vi "MultiOpto_Host.vi"() -> ()   [LabVIEW 2018]
uses:
  <instrlib>/niDMM/nidmm.llb/niDMM Resolution in Digits.ctl
  <instrlib>/niDMM/nidmm.llb/niDMM Function.ctl
  <instrlib>/niDCPower/nidcpower.llb/niDCPower Measurement Type.ctl
  <instrlib>/niDMM/nidmm.llb/niDMM Configure Measurement Digits.vi
  <instrlib>/niScope/Configure/Trigger/niScope Configure Trigger Window.vi
  <instrlib>/niScope/Acquire/Fetch/niScope Multi Fetch Cluster.vi
  <instrlib>/niScope/Acquire/Fetch/niScope Fetch.vi
panel:
  in  "Full Log Path":path=path "D:/NI LabVIEW/MultiOpto/Full Log"
  in  "Full Log Wait":u32=200
  in  "NI DMM 1":refnum<k15>="PXI1Slot6_3"
  in  "NI DMM 2":refnum<k15>="PXI1Slot6_3"
  in  "Ophir 2 Tab":enum32{"Ophir 2", "System Panel"}(tab)
  out "Ophir 2 Initialization":bool caption="Initialization"
  in  "Ophir 2 Clear":bool caption="Clear"
  out "Ophir 2 MAX":dbl caption="MAX" format="%#_4g"
  out "Ophir 2 Optical Power":dbl caption="Optical Power" format="%#_4g"
  out "Ophir 2 Over Range":bool caption="Over Range"
  out "Ophir 2 Char":dbl(graph)=6.67426339573744e-05
  in  "Ophir 2 units":string(combo)="1000" caption="Units"
  in  "Ophir 2 Info":u16(ring)=1 caption="Info" items=["Device : JUNO; s/n:903794", "Head : PD300-IRG-v1; s/n:908004"]
  in  "Ophir 2 Wait":u32=100 caption="Wait"
  out "Ophir 2 error out":errorcluster caption="error out"
  out "Ophir 2 dup Visa Session":refnum<visa-resource-name>="USB0::0x0BD3::0x0777::NI-VISA-10003::RAW" caption="dup Visa Session"
  in  "Ophir 2 GPIB Address (10)":string="10" caption="GPIB Address (10)"
  in  "Ophir 2 Select Communication Protocol":u16(ring) caption="Select Communication Protocol" items=["USB", "RS232", "GPIB"]
  in  "Ophir 2 usb channel":i16 caption="usb channel"
  in  "Ophir 2 Baud Rate (3:9600)":i16(ring)=3 caption="Baud Rate (3:9600)" items=["300", "1200", "4800", "9600", "19200", "38400"]
  in  "Ophir 2 Port Number (default 2)":i16=2 caption="Port Number (default 2)" min=0 max=20
  in  "Ophir 2 error in (no error)":errorcluster caption="error in (no error)"
  out "Ophir 2 Status":bool caption="Status"
  out "Ophir 2 Real Optical Power":dbl format="%.3e"
  in  "Ophir 1 Tab":enum32{"Ophir 1", "System Panel"}(tab)
  out "Ophir 1 Initialization":bool caption="Initialization"
  in  "Ophir 1 units":string(combo)="1000" caption="Units"
  out "Ophir 1 Char":dbl(graph)=6.67426339573744e-05
  out "Ophir 1 Over Range":bool caption="Over Range"
  out "Ophir 1 Optical Power":dbl caption="Optical Power" format="%#_4g"
  out "Ophir 1 MAX":dbl caption="MAX" format="%#_4g"
  in  "Ophir 1 Clear":bool caption="Clear"
  in  "Ophir 1 Info":u16(ring)=1 caption="Info" items=["Device : JUNO; s/n:903795", "Head : PD300R-IR   ; s/n:873888"]
  in  "Ophir 1 Wait":u32=100 caption="Wait"
  in  "Ophir 1 error in (no error)":errorcluster caption="error in (no error)"
  out "Ophir 1 error out":errorcluster caption="error out"
  in  "Ophir 1 Select Communication Protocol":u16(ring) caption="Select Communication Protocol" items=["USB", "RS232", "GPIB"]
  in  "Ophir 1 usb channel":i16 caption="usb channel"
  in  "Ophir 1 Port Number (default 2)":i16=1 caption="Port Number (default 2)" min=0 max=20
  in  "Ophir 1 Baud Rate (3:9600)":i16(ring)=3 caption="Baud Rate (3:9600)" items=["300", "1200", "4800", "9600", "19200", "38400"]
  in  "Ophir 1 GPIB Address (10)":string="10" caption="GPIB Address (10)"
  out "Ophir 1 dup Visa Session":refnum<visa-resource-name>="USB0::0x0BD3::0x0777::NI-VISA-10003::RAW" caption="dup Visa Session"
  out "Ophir 1 Status":bool caption="Status"
  out "Ophir 1 Real Optical Power":dbl format="%.3e"
  out "Образец №":string
  in  "NI DMM 2 Tab":enum32{"Ampermeter", "Ohmmeter", "System Panel"}(tab)
  out "NI DMM 2 Current":dbl caption="Current" format="%_4g"
  out "NI DMM 2 Current Char":dbl(graph)=6.67426339573744e-05
  in  "NI DMM 2 Ampermeter path":path=path "D:/NI LabVIEW/MultiOpto/NI DMM 2" caption="NI DMM 2 Path"
  in  "NI DMM 2 units":string(combo)="1" caption="Units"
  in  "NI DMM 2 Current Range":string(combo)="-1" caption="Range"
  in  "NI DMM 2 Current Wait":u32=100 caption="Wait"
  in  "NI DMM 2 Ohmmeter path":path=path "D:/NI LabVIEW/MultiOpto/NI DMM 2" caption="Ohmmeter Path"
  out "NI DMM 2 Resistance":dbl caption="Resistance" format="%_4g"
  out "NI DMM 2 Resistance Char":dbl(graph)=6.67426339573744e-05
  in  "NI DMM 2 Resistance units":string(combo)="1" caption="Units"
  in  "NI DMM 2 Resistance Range":string(combo)="-1" caption="Range"
  in  "NI DMM 2 Resistance Wait":u32=100 caption="Wait"
  out "NI DMM 2 Status":bool
  out "NI DMM 2 Current output file":refnum<file>
  out "NI DMM 2error out":errorcluster
  in  "NI DMM 2 error in":errorcluster
  out "NI DMM 2 Option Return":enum32{"Ampermeter button", "Ohmmeter button"}(ring)
  out "NI DMM 2 Resistance output file":refnum<file>
  in  "NI DMM 1 Tab":enum32{"Ampermeter", "Ohmmeter", "System Panel"}(tab)
  out "NI DMM 1 Current Char":dbl(graph)=6.67426339573744e-05
  out "NI DMM 1 Current":dbl caption="Current" format="%_4g"
  in  "NI DMM 1 Ampermeter path":path=path "D:/NI LabVIEW/MultiOpto/NI DMM 1" caption="Ampermeter Path"
  in  "NI DMM 1 units":string(combo)="1" caption="Units"
  in  "NI DMM 1 Current Range":string(combo)="-1" caption="Range"
  in  "NI DMM 1 Current Wait":u32=100 caption="Wait"
  in  "NI DMM 1 Ohmmeter path":path=path "D:/NI LabVIEW/MultiOpto/NI DMM 1" caption="Ohmmeter Path"
  out "NI DMM 1 Resistance":dbl caption="Resistance" format="%_6g"
  out "NI DMM 1 Resistance Char":dbl(graph)=6.67426339573744e-05
  in  "NI DMM 1 Resistance units":string(combo)="1" caption="Units"
  in  "NI DMM 1 Resistance Range":string(combo)="-1" caption="Range"
  in  "NI DMM 1 Resistance Wait":u32=100 caption="Wait"
  out "NI DMM 1 Status":bool
  out "NI DMM 1 Current output file":refnum<file>
  out "NI DMM 1 error out":errorcluster
  in  "NI DMM 1 error in":errorcluster
  out "NI DMM 1 Option Return":enum32{"Ampermeter button", "Ohmmeter button"}(ring)
  out "NI DMM 1 Resistance output file":refnum<file>
  out "SEL":bool
  out "SEU":bool caption="SEL"
  in  "NI Scope Tab":enum32{"NI Scope", "System Panel"}(tab)
  in  "vertical range":dbl=2.0 caption="Vertical Range" format="%.2f"
  out "SEU Last Level":dbl
  out "RealTime Waveform":T1(graph) caption="PC_MON Waveform"
  out "SEU Waveform":T1(graph) caption="SHUTDOWN Waveform"
  out "SEU_Counter":u32 caption="SEU counter"
  out "SEU_warning":bool caption="Find SEL"
  in  "Low Level":dbl=0.35 format="%.2f"
  in  "High Level":dbl=0.65 format="%.2f"
  in  "NI Scope":refnum<k15>="PXI1Slot5_2" caption="Scope"
  in  "AC/DC/Groun":i32(ring)=1 items=["AC", "DC", "Ground"]
  in  "Trigger Source":string(combo)="0"
  in  "SEU path":path=path "D:/NI LabVIEW/MultiOpto/SEU" caption="SEU Path"
  in  "Channel for SEU":T2(radio)
  out "SEU output file refnum":refnum<file>
  out "NI Scope Status":bool
  out "NI Scope error out":errorcluster
  in  "NI Scope error in":errorcluster
  in  "STOP":bool
  in  "DC Power Tab":enum32{"DC-Power", "System Panel"}(tab)
  out "P2 CH1_warning":bool caption="VCC_warning"
  out "P2 CH1_counter":u32 caption="VCC_counter"
  in  "P2 CH1_selcur, A":dbl=0.2 caption="current limit" format="%_6p"
  in  "P2 CH1 Used":bool
  in  "P2 CH1":bool
  out "P2 CH1_char":dbl(graph)=4.1881856349625015e-07
  in  "P2 CH1, V":dbl=4.9 caption="voltage level" format="%_6p"
  out "P2 CH1_cur, A":dbl caption="measurement" format="%_6g"
  in  "P2 CH1_curlim, A":dbl=0.015 caption="current limit" format="%_6p"
  in  "P1 CH0_selcur, A":dbl=0.2 caption="current limit" format="%_6p"
  in  "P1 CH1_selcur, A":dbl=0.2 caption="current limit" format="%_6p"
  in  "P2 CH0_selcur, A":dbl=0.2 caption="current limit" format="%_6p"
  out "P2 CH0_counter":u32 caption="VCC_counter"
  out "P2 CH0_warning":bool caption="VCC_warning"
  out "P1 CH1_counter":u32 caption="VCC_counter"
  out "P1 CH1_warning":bool caption="VCC_warning"
  out "P1 CH0_counter":u32 caption="VCC_counter"
  out "P1 CH0_warning":bool caption="VCC_warning"
  in  "P2 CH0":bool
  in  "P1 CH1":bool
  in  "P1 CH0":bool
  in  "P2 CH0_curlim, A":dbl=0.015 caption="current limit" format="%_6p"
  out "P2 CH0_cur, A":dbl caption="measurement" format="%_6g"
  in  "P2 CH0, V":dbl=2.5 caption="voltage level" format="%_6p"
  out "P2 CH0_char":dbl(graph)=8.408429577071082e-05
  in  "P1 CH1_curlim, A":dbl=0.015 caption="current limit" format="%_6p"
  out "P1CH1_cur, A":dbl caption="measurement" format="%_6g"
  in  "P1 CH1, V":dbl=2.5 caption="voltage level" format="%_6p"
  out "P1 CH1_char":dbl(graph)=6.336785656464814e-07
  in  "P1 CH0_curlim, A":dbl=0.015 caption="current limit" format="%_6p"
  out "P1 CH0_cur, A":dbl caption="measurement" format="%_6g"
  in  "P1 CH0, V":dbl=2.5 caption="voltage level" format="%_6p"
  out "P1 CH0_char":dbl(graph)=8.030591065176734e-05
  in  "POWER 2 (CH0, CH1)":refnum<k15>="PXI1Slot3_3" caption="PRBS"
  in  "POWER 1 (CH0, CH1)":refnum<k15>="PXI1Slot2_2" caption="VСС_+5"
  in  "P1 CH0 Used":bool
  in  "P2 CH0 Used":bool
  in  "P1 CH1 Used":bool
  in  "SIM_SEL":bool
  in  "SEL Time Cycle":u32=100
  in  "SEL path":path=path "D:/NI LabVIEW/MultiOpto/SEL" caption="SEL Path"
  out "Power OFF":bool
  in  "Считать SIM_SEL":bool
  out "Ready Status":bool
  out "DC Power 2 error out":errorcluster
  out "DC Power 1 error out":errorcluster
  out "SEL output file refnum":refnum<file>
  # "Че там?"
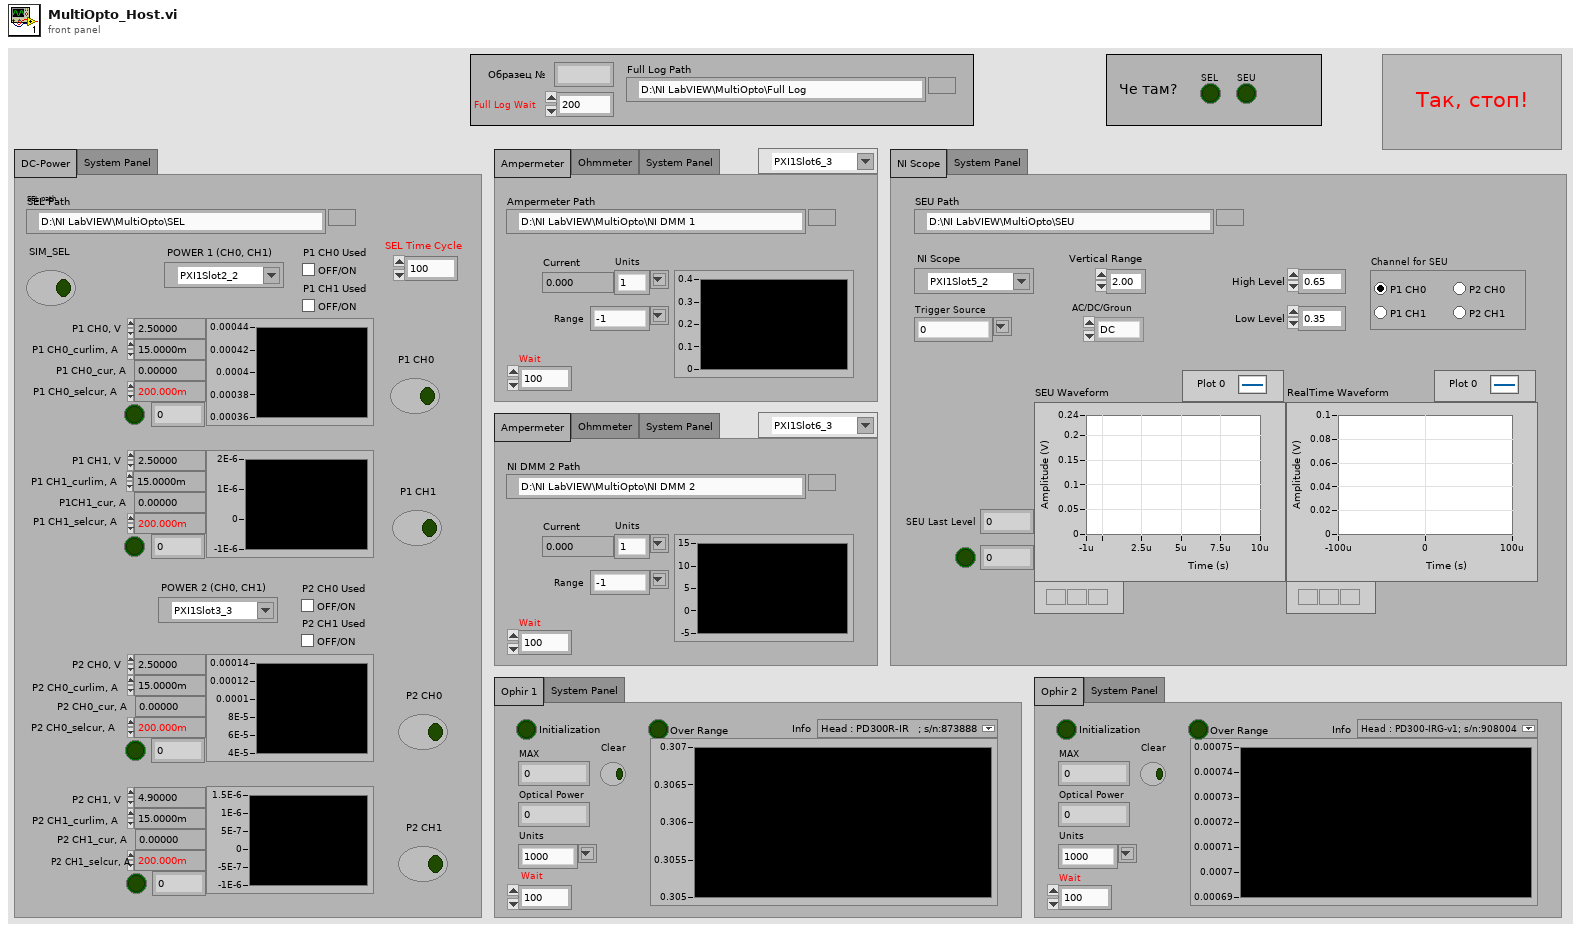
[diagram p1: front panel]
types:
  T1 = cluster{"relativeInitialX":dbl, "xIncrement":dbl, "wfm":dbl[]}[]
  T2 = enum32{"Radio Selection P1 CH0", "Radio Selection P1 CH1", "Radio Selection P2 CH0", "Radio Selection P2 CH1"}
  T3 = enum8{"Enabled", "Disabled", "Disabled and Grayed Out"}
  T4 = enum16{"open", "replace", "create", "open or create", "replace or create", "replace or create with confirmation"}
  T5 = typedef "niDMM Function.ctl" = enum16{"DC Volts", "AC Volts", "DC Current", "AC Current", "2-wire Resistance", "4-wire Resistance", "Diode", "Frequency", "Period", "AC Volts DC Coupled", "Capacitance", "Inductance", "Temperature"}
  T6 = typedef "niDMM Resolution in Digits.ctl" = dbl
  T7 = typedef "niDCPower Measurement Type.ctl" = i32
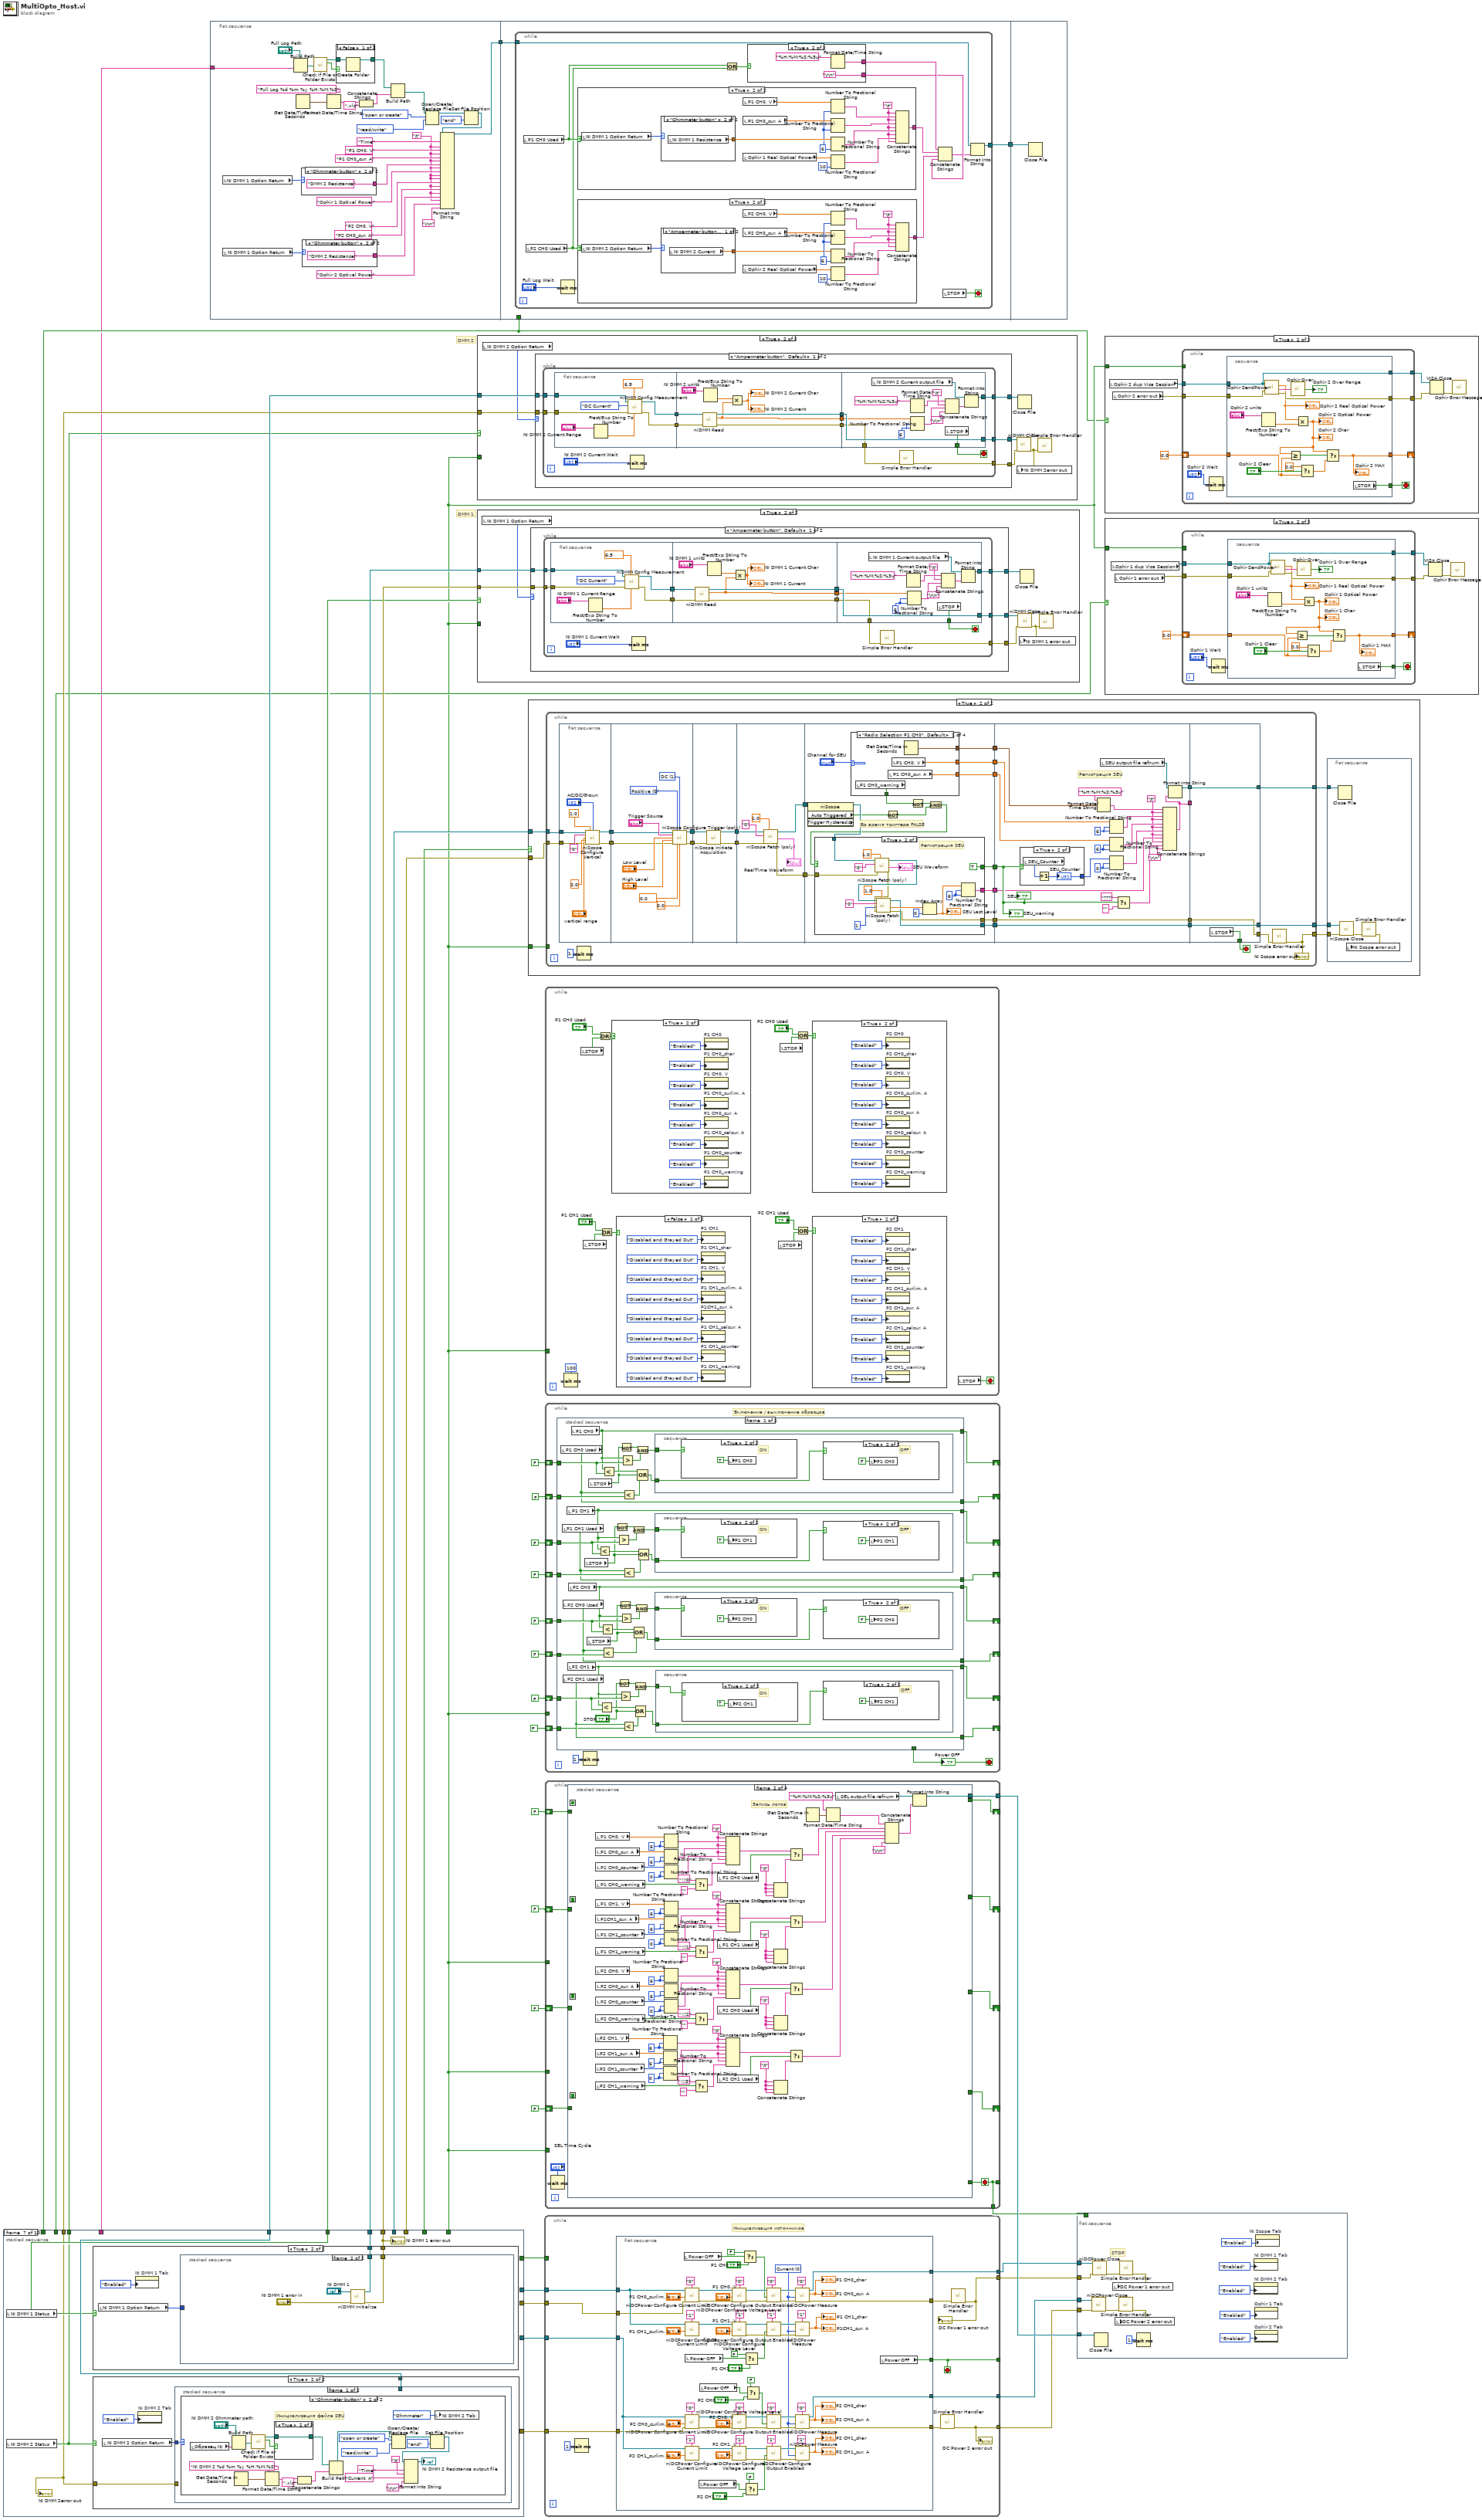
[diagram p0: block diagram]
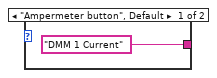
[diagram p2: hidden frame]
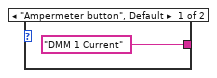
[diagram p3: hidden frame]
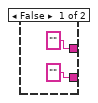
[diagram p5: hidden frame]
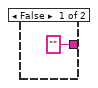
[diagram p6: hidden frame]
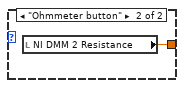
[diagram p7: hidden frame]
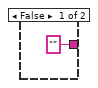
[diagram p8: hidden frame]
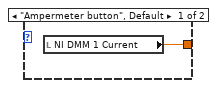
[diagram p9: hidden frame]
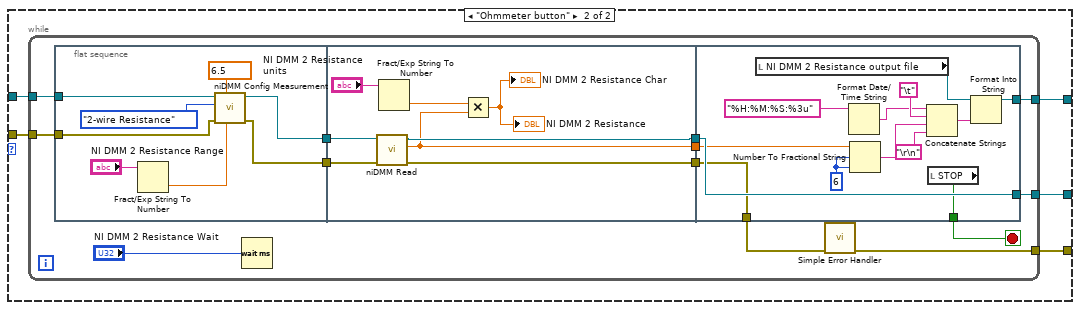
[diagram p13: hidden frame]
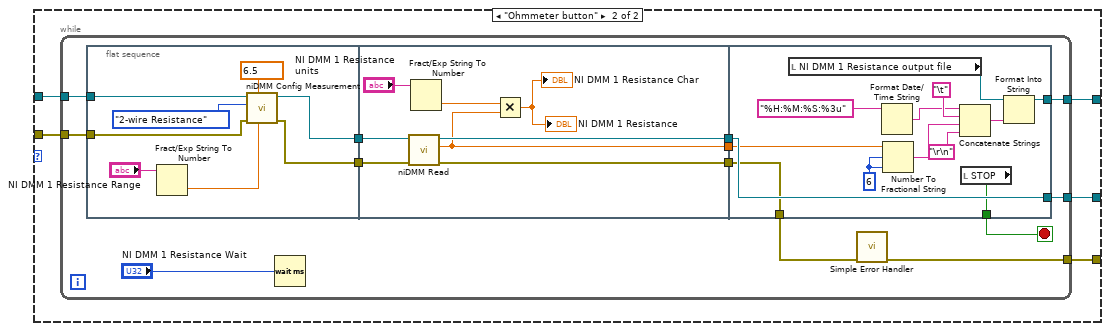
[diagram p15: hidden frame]
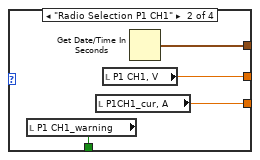
[diagram p17: hidden frame]
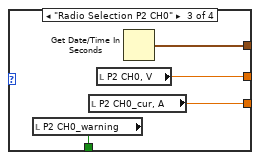
[diagram p18: hidden frame]
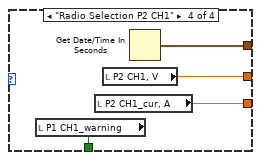
[diagram p19: hidden frame]
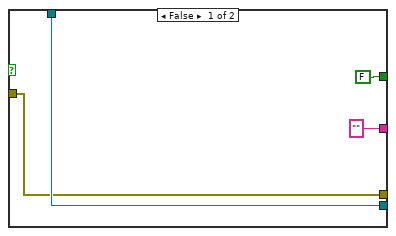
[diagram p20: hidden frame]
diagram:
  # "DMM 2"
  # "DMM 1"
  n1 = stacked-sequence {
    tunnel: [_ _ _ _ w165 _ _ _ _ _] -> w23
    tunnel: [_ _ _ _ w164 _ _ _ _ _] -> w22
    tunnel: [_ _ _ _ w163 _ _ _ _ _] -> w18
    tunnel: [_ _ _ _ w162 _ _ _ _ _] -> w17
    tunnel: [_ _ _ _ _ _ _ _ _ w412] -> w16
    tunnel: [_ _ _ _ _ _ _ _ _ w412] -> w3
    tunnel: [_ _ _ _ _ w178 _ _ _ _] -> w15
    tunnel: [_ _ _ _ _ _ w234 _ _ _] -> w14
    tunnel: [_ _ _ _ _ _ w237 _ _ _] -> w13
    tunnel: [_ _ _ _ _ w177 _ _ _ _] -> w12
    tunnel: [_ _ _ _ _ _ w233 _ _ _] -> w11
    tunnel: [_ _ _ _ _ _ w232 _ _ _] -> w10
    tunnel: [_ _ _ _ _ w176 _ _ _ _] -> w9
    tunnel: [_ _ _ _ _ _ w236 _ _ _] -> w8
    tunnel: [_ _ _ _ _ _ w235 _ _ _] -> w7
    tunnel: [_ _ _ _ _ _ _ w366 _ _] -> w6
    tunnel: [_ _ _ _ _ _ _ _ w389 _] -> w2
    tunnel: [_ _ w114 _ _ _ _ _ _ _] -> w1
    frame #0 {
      w39 = FALSE
      w41 = FALSE ("NI Scope Status")
      w44 = u32 0 ("SEU_Counter")
      w40 = FALSE ("STOP")
      # "Начальная конфигурация переменных"
      n2 = local write "Ophir 2 Over Range"(w39) -> ()
      n3 = local write "Ophir 1 Over Range"(w39) -> ()
      n4 = local write "Ophir 1 Initialization"(w39) -> ()
      n5 = local write "Ophir 2 Initialization"(w39) -> ()
      n6 = local write "Ophir 1 Clear"(w39) -> ()
      n7 = local write "Ophir 2 Clear"(w39) -> ()
      n8 = local write "STOP"(w40) -> ()
      n9 = local write "P1 CH0"(w40) -> ()
      n10 = local write "P1 CH1"(w40) -> ()
      n11 = local write "P2 CH0"(w40) -> ()
      n12 = local write "P2 CH1"(w40) -> ()
      n13 = local write "Power OFF"(w40) -> ()
      n14 = local write "P1 CH0 Used"(w40) -> ()
      n15 = local write "P1 CH1 Used"(w40) -> ()
      n16 = local write "P2 CH0 Used"(w40) -> ()
      n17 = local write "P2 CH1 Used"(w40) -> ()
      n18 = local write "Считать SIM_SEL"(w40) -> ()
      n19 = local write "SEL"(w40) -> ()
      n20 = local write "SEU"(w40) -> ()
      n21 = local write "SEU_warning"(w40) -> ()
      n22 = local write "P1 CH0_warning"(w40) -> ()
      n23 = local write "P1 CH1_warning"(w40) -> ()
      n24 = local write "P2 CH0_warning"(w40) -> ()
      n25 = local write "P2 CH1_warning"(w40) -> ()
      n26 = local write "SEU_warning"(w40) -> ()
      n27 = local write "SEU Last Level"(0.0 ("SEU Level")) -> ()
      n28 = local write "SEU_Counter"(w44) -> ()
      n29 = local write "P1 CH0_counter"(w44) -> ()
      n30 = local write "P1 CH1_counter"(w44) -> ()
      n31 = local write "P2 CH0_counter"(w44) -> ()
      n32 = local write "P2 CH1_counter"(w44) -> ()
      n33 = local write "Образец №"("" ("Образец №")) -> ()
      n34 = local write "Ready Status"(FALSE ("Ready Status")) -> ()
      n35 = local write "NI Scope Status"(w41) -> ()
      n36 = local write "NI DMM 2 Status"(w41) -> ()
      n37 = local write "NI DMM 1 Status"(w41) -> ()
      n38 = local write "Ophir 1 Status"(w41) -> ()
      n39 = local write "Ophir 2 Status"(w41) -> ()
    }
    frame #1 {
      n40 = stacked-sequence {
        frame #0 {
          n41 = local read "P1 CH0 Used"() -> (w46:bool)
          n42 = case shown="False" w46 {
            frame False {
              n43 = property on="P1 CH0" class="Bool (strict)"("DisabledEnum"=T3."Disabled and Grayed Out" ("Disabled")) -> ()  [unwired: 2 in, 2 out]
              n44 = property on="P1 CH0_char" class="WFChart (strict)"("DisabledEnum"=T3."Disabled and Grayed Out" ("Disabled")) -> ()  [unwired: 2 in, 2 out]
              n45 = property on="P1 CH0, V" class="DigNum (strict)"("DisabledEnum"=T3."Disabled and Grayed Out" ("Disabled")) -> ()  [unwired: 2 in, 2 out]
              n46 = property on="P1 CH0_curlim, A" class="DigNum (strict)"("DisabledEnum"=T3."Disabled and Grayed Out" ("Disabled")) -> ()  [unwired: 2 in, 2 out]
              n47 = property on="P1 CH0_cur, A" class="DigNum (strict)"("DisabledEnum"=T3."Disabled and Grayed Out" ("Disabled")) -> ()  [unwired: 2 in, 2 out]
              n48 = property on="P1 CH0_selcur, A" class="DigNum (strict)"("DisabledEnum"=T3."Disabled and Grayed Out" ("Disabled")) -> ()  [unwired: 2 in, 2 out]
              n49 = property on="P1 CH0_counter" class="DigNum (strict)"("DisabledEnum"=T3."Disabled and Grayed Out" ("Disabled")) -> ()  [unwired: 2 in, 2 out]
              n50 = property on="P1 CH0_warning" class="Bool (strict)"("DisabledEnum"=T3."Disabled and Grayed Out" ("Disabled")) -> ()  [unwired: 2 in, 2 out]
            }
            frame True {
              n51 = property on="P1 CH0" class="Bool (strict)"("DisabledEnum"=T3."Enabled" ("Disabled")) -> ()  [unwired: 2 in, 2 out]
              n52 = property on="P1 CH0_char" class="WFChart (strict)"("DisabledEnum"=T3."Enabled" ("Disabled")) -> ()  [unwired: 2 in, 2 out]
              n53 = property on="P1 CH0, V" class="DigNum (strict)"("DisabledEnum"=T3."Enabled" ("Disabled")) -> ()  [unwired: 2 in, 2 out]
              n54 = property on="P1 CH0_curlim, A" class="DigNum (strict)"("DisabledEnum"=T3."Enabled" ("Disabled")) -> ()  [unwired: 2 in, 2 out]
              n55 = property on="P1 CH0_cur, A" class="DigNum (strict)"("DisabledEnum"=T3."Enabled" ("Disabled")) -> ()  [unwired: 2 in, 2 out]
              n56 = property on="P1 CH0_selcur, A" class="DigNum (strict)"("DisabledEnum"=T3."Enabled" ("Disabled")) -> ()  [unwired: 2 in, 2 out]
              n57 = property on="P1 CH0_counter" class="DigNum (strict)"("DisabledEnum"=T3."Enabled" ("Disabled")) -> ()  [unwired: 2 in, 2 out]
              n58 = property on="P1 CH0_warning" class="Bool (strict)"("DisabledEnum"=T3."Enabled" ("Disabled")) -> ()  [unwired: 2 in, 2 out]
            }
          }
        }
        frame #1 {
          n59 = local read "P1 CH1 Used"() -> (w63:bool)
          n60 = case shown="False" w63 {
            frame False {
              n61 = property on="P1 CH1" class="Bool (strict)"("DisabledEnum"=T3."Disabled and Grayed Out" ("Disabled")) -> ()  [unwired: 2 in, 2 out]
              n62 = property on="P1 CH1_char" class="WFChart (strict)"("DisabledEnum"=T3."Disabled and Grayed Out" ("Disabled")) -> ()  [unwired: 2 in, 2 out]
              n63 = property on="P1 CH1, V" class="DigNum (strict)"("DisabledEnum"=T3."Disabled and Grayed Out" ("Disabled")) -> ()  [unwired: 2 in, 2 out]
              n64 = property on="P1 CH1_curlim, A" class="DigNum (strict)"("DisabledEnum"=T3."Disabled and Grayed Out" ("Disabled")) -> ()  [unwired: 2 in, 2 out]
              n65 = property on="P1CH1_cur, A" class="DigNum (strict)"("DisabledEnum"=T3."Disabled and Grayed Out" ("Disabled")) -> ()  [unwired: 2 in, 2 out]
              n66 = property on="P1 CH1_selcur, A" class="DigNum (strict)"("DisabledEnum"=T3."Disabled and Grayed Out" ("Disabled")) -> ()  [unwired: 2 in, 2 out]
              n67 = property on="P1 CH1_counter" class="DigNum (strict)"("DisabledEnum"=T3."Disabled and Grayed Out" ("Disabled")) -> ()  [unwired: 2 in, 2 out]
              n68 = property on="P1 CH1_warning" class="Bool (strict)"("DisabledEnum"=T3."Disabled and Grayed Out" ("Disabled")) -> ()  [unwired: 2 in, 2 out]
            }
            frame True {
              n69 = property on="P1 CH1" class="Bool (strict)"("DisabledEnum"=T3."Enabled" ("Disabled")) -> ()  [unwired: 2 in, 2 out]
              n70 = property on="P1 CH1_char" class="WFChart (strict)"("DisabledEnum"=T3."Enabled" ("Disabled")) -> ()  [unwired: 2 in, 2 out]
              n71 = property on="P1 CH1, V" class="DigNum (strict)"("DisabledEnum"=T3."Enabled" ("Disabled")) -> ()  [unwired: 2 in, 2 out]
              n72 = property on="P1 CH1_curlim, A" class="DigNum (strict)"("DisabledEnum"=T3."Enabled" ("Disabled")) -> ()  [unwired: 2 in, 2 out]
              n73 = property on="P1CH1_cur, A" class="DigNum (strict)"("DisabledEnum"=T3."Enabled" ("Disabled")) -> ()  [unwired: 2 in, 2 out]
              n74 = property on="P1 CH1_selcur, A" class="DigNum (strict)"("DisabledEnum"=T3."Enabled" ("Disabled")) -> ()  [unwired: 2 in, 2 out]
              n75 = property on="P1 CH1_counter" class="DigNum (strict)"("DisabledEnum"=T3."Enabled" ("Disabled")) -> ()  [unwired: 2 in, 2 out]
              n76 = property on="P1 CH1_warning" class="Bool (strict)"("DisabledEnum"=T3."Enabled" ("Disabled")) -> ()  [unwired: 2 in, 2 out]
            }
          }
        }
        frame #2 {
          n77 = local read "P2 CH0 Used"() -> (w80:bool)
          n78 = case shown="False" w80 {
            frame False {
              n79 = property on="P2 CH0" class="Bool (strict)"("DisabledEnum"=T3."Disabled and Grayed Out" ("Disabled")) -> ()  [unwired: 2 in, 2 out]
              n80 = property on="P2 CH0_char" class="WFChart (strict)"("DisabledEnum"=T3."Disabled and Grayed Out" ("Disabled")) -> ()  [unwired: 2 in, 2 out]
              n81 = property on="P2 CH0, V" class="DigNum (strict)"("DisabledEnum"=T3."Disabled and Grayed Out" ("Disabled")) -> ()  [unwired: 2 in, 2 out]
              n82 = property on="P2 CH0_curlim, A" class="DigNum (strict)"("DisabledEnum"=T3."Disabled and Grayed Out" ("Disabled")) -> ()  [unwired: 2 in, 2 out]
              n83 = property on="P2 CH0_cur, A" class="DigNum (strict)"("DisabledEnum"=T3."Disabled and Grayed Out" ("Disabled")) -> ()  [unwired: 2 in, 2 out]
              n84 = property on="P2 CH0_selcur, A" class="DigNum (strict)"("DisabledEnum"=T3."Disabled and Grayed Out" ("Disabled")) -> ()  [unwired: 2 in, 2 out]
              n85 = property on="P2 CH0_counter" class="DigNum (strict)"("DisabledEnum"=T3."Disabled and Grayed Out" ("Disabled")) -> ()  [unwired: 2 in, 2 out]
              n86 = property on="P2 CH0_warning" class="Bool (strict)"("DisabledEnum"=T3."Disabled and Grayed Out" ("Disabled")) -> ()  [unwired: 2 in, 2 out]
            }
            frame True {
              n87 = property on="P2 CH0" class="Bool (strict)"("DisabledEnum"=T3."Enabled" ("Disabled")) -> ()  [unwired: 2 in, 2 out]
              n88 = property on="P2 CH0_char" class="WFChart (strict)"("DisabledEnum"=T3."Enabled" ("Disabled")) -> ()  [unwired: 2 in, 2 out]
              n89 = property on="P2 CH0, V" class="DigNum (strict)"("DisabledEnum"=T3."Enabled" ("Disabled")) -> ()  [unwired: 2 in, 2 out]
              n90 = property on="P2 CH0_curlim, A" class="DigNum (strict)"("DisabledEnum"=T3."Enabled" ("Disabled")) -> ()  [unwired: 2 in, 2 out]
              n91 = property on="P2 CH0_cur, A" class="DigNum (strict)"("DisabledEnum"=T3."Enabled" ("Disabled")) -> ()  [unwired: 2 in, 2 out]
              n92 = property on="P2 CH0_selcur, A" class="DigNum (strict)"("DisabledEnum"=T3."Enabled" ("Disabled")) -> ()  [unwired: 2 in, 2 out]
              n93 = property on="P2 CH0_counter" class="DigNum (strict)"("DisabledEnum"=T3."Enabled" ("Disabled")) -> ()  [unwired: 2 in, 2 out]
              n94 = property on="P2 CH0_warning" class="Bool (strict)"("DisabledEnum"=T3."Enabled" ("Disabled")) -> ()  [unwired: 2 in, 2 out]
            }
          }
        }
        frame #3 {
          n95 = local read "P2 CH1 Used"() -> (w97:bool)
          n96 = case shown="False" w97 {
            frame False {
              n97 = property on="P2 CH1" class="Bool (strict)"("DisabledEnum"=T3."Disabled and Grayed Out" ("Disabled")) -> ()  [unwired: 2 in, 2 out]
              n98 = property on="P2 CH1_char" class="WFChart (strict)"("DisabledEnum"=T3."Disabled and Grayed Out" ("Disabled")) -> ()  [unwired: 2 in, 2 out]
              n99 = property on="P2 CH1, V" class="DigNum (strict)"("DisabledEnum"=T3."Disabled and Grayed Out" ("Disabled")) -> ()  [unwired: 2 in, 2 out]
              n100 = property on="P2 CH1_curlim, A" class="DigNum (strict)"("DisabledEnum"=T3."Disabled and Grayed Out" ("Disabled")) -> ()  [unwired: 2 in, 2 out]
              n101 = property on="P2 CH1_cur, A" class="DigNum (strict)"("DisabledEnum"=T3."Disabled and Grayed Out" ("Disabled")) -> ()  [unwired: 2 in, 2 out]
              n102 = property on="P2 CH1_selcur, A" class="DigNum (strict)"("DisabledEnum"=T3."Disabled and Grayed Out" ("Disabled")) -> ()  [unwired: 2 in, 2 out]
              n103 = property on="P2 CH1_counter" class="DigNum (strict)"("DisabledEnum"=T3."Disabled and Grayed Out" ("Disabled")) -> ()  [unwired: 2 in, 2 out]
              n104 = property on="P2 CH1_warning" class="Bool (strict)"("DisabledEnum"=T3."Disabled and Grayed Out" ("Disabled")) -> ()  [unwired: 2 in, 2 out]
            }
            frame True {
              n105 = property on="P2 CH1" class="Bool (strict)"("DisabledEnum"=T3."Enabled" ("Disabled")) -> ()  [unwired: 2 in, 2 out]
              n106 = property on="P2 CH1_char" class="WFChart (strict)"("DisabledEnum"=T3."Enabled" ("Disabled")) -> ()  [unwired: 2 in, 2 out]
              n107 = property on="P2 CH1, V" class="DigNum (strict)"("DisabledEnum"=T3."Enabled" ("Disabled")) -> ()  [unwired: 2 in, 2 out]
              n108 = property on="P2 CH1_curlim, A" class="DigNum (strict)"("DisabledEnum"=T3."Enabled" ("Disabled")) -> ()  [unwired: 2 in, 2 out]
              n109 = property on="P2 CH1_cur, A" class="DigNum (strict)"("DisabledEnum"=T3."Enabled" ("Disabled")) -> ()  [unwired: 2 in, 2 out]
              n110 = property on="P2 CH1_selcur, A" class="DigNum (strict)"("DisabledEnum"=T3."Enabled" ("Disabled")) -> ()  [unwired: 2 in, 2 out]
              n111 = property on="P2 CH1_counter" class="DigNum (strict)"("DisabledEnum"=T3."Enabled" ("Disabled")) -> ()  [unwired: 2 in, 2 out]
              n112 = property on="P2 CH1_warning" class="Bool (strict)"("DisabledEnum"=T3."Enabled" ("Disabled")) -> ()  [unwired: 2 in, 2 out]
            }
          }
        }
      }
    }
    frame #2 {
      n113 = call "MultiOpto_Begin.vi"() -> ("NI DMM 2 Status"=→"NI DMM 2 Status":bool, "NI DMM 1 Status"=→"NI DMM 1 Status":bool, "Ophir 2 Status"=→"Ophir 2 Status":bool, "Ophir 1 Status"=→"Ophir 1 Status":bool, "Текущий Образец №"=w114:string, "NI Scope Status"=→"NI Scope Status":bool, "NI DMM 2 option return"=→"NI DMM 2 Option Return":enum32{"Ampermeter button", "Ohmmeter button"}, "NI DMM 1 option return"=→"NI DMM 1 Option Return":enum32{"Ampermeter button", "Ohmmeter button"})  [unwired: 2 in]
      "Образец №" <- w114
    }
    frame #3 {
      w124 = "\t"
      # "Инициализация файла SEL"
      n114 = local read "Образец №"() -> (w143:string)
      n115 = Build Path(base path="SEL path", name or relative path=w143) -> (appended path=w158:path)
      n116 = Get Date/Time In Seconds() -> (seconds since 1Jan1904=w154:timestamp)
      n117 = call <vilib>:"Check if File or Folder Exists.vi"("path"=w158) -> ("file or folder exists?"=w157:bool, "dup path"=w156:path)  [unwired: 8 in, 1 out]
      n118 = Format Date/Time String(time format string (%c)="SEL %d %m %y %H.%M.%S", seconds (now)=w154) -> (date/time string=w153:string)  [unwired: 1 in]
      n119 = case shown="True" w157 {
        tunnel: w156 -> [w160 w161]
        tunnel: [w159 w161] -> w155
        frame False {
          n120 = Create Folder(path (use dialog)=w160) -> (created path=w159:path)  [unwired: 2 in, 2 out]
        }
        frame True {
        }
      }
      n121 = Concatenate Strings(w153, ".xls" ("string")) -> (w150:string)
      n122 = Build Path(base path=w155, name or relative path=w150) -> (appended path=w147:path)
      n123 = Open/Create/Replace File(file path (use dialog)=w147, operation (0:open)=T4."open or create", access (0:read/write)=enum16{"read/write", "read-only", "write-only"}."read/write") -> (refnum out=w146:refnum<file>)  [unwired: 3 in, 2 out]
      n124 = Set File Position(refnum=w146, from (0:start)=enum16{"start", "end", "current"}."end") -> (refnum out=w125:refnum<file>)  [unwired: 2 in, 1 out]
      n125 = Format Into String(initial string=w125, "Time" ("string"), w124, "P1 CH0, V" ("string"), w124, "P1 CH0_cur, A" ("string"), w124, "P1 CH0_counter" ("string"), w124, "!!!0" ("input 7"), w124, "P1 CH1, V" ("string"), w124, "P1 CH1_cur, A" ("string"), w124, "P1 CH1_counter" ("string"), w124, "!!!1" ("input 7"), w124, "P2 CH0, V" ("string"), w124, "P2 CH0_cur, A" ("string"), w124, "P2 CH0_counter" ("string"), w124, "!!!2" ("input 7"), w124, "P2 CH1, V" ("string"), w124, "P2 CH1_cur, A" ("string"), w124, "P2 CH1_counter" ("string"), "!!!3" ("input 7"), "\r\n") -> (resulting string=→"SEL output file refnum":refnum<file>)  [unwired: 2 in, 1 out]
    }
    frame #4 {
      # "Инициализация источника"
      n126 = call <instrlib>:"niDCPower Initialize.vi"("resource name"="POWER 1 (CH0, CH1)") -> ("error out"=w174:errorcluster, "instrument handle out"=w175:refnum<k15>)  [unwired: 3 in, 6 out]
      n127 = call <instrlib>:"niDCPower Initialize.vi"("resource name"="POWER 2 (CH0, CH1)") -> ("error out"=w171:errorcluster, "instrument handle out"=w172:refnum<k15>)  [unwired: 3 in, 6 out]
      n128 = call <instrlib>:"niDCPower Configure Voltage Level.vi"("error in (no error)"=w174, "voltage level"=0.0, "channel name"="0,1", "instrument handle"=w175) -> ("error out"=w163:errorcluster, "instrument handle out"=w165:refnum<k15>)  [unwired: 6 in]
      n129 = call <instrlib>:"niDCPower Configure Voltage Level.vi"("error in (no error)"=w171, "voltage level"=0.0, "channel name"="0,1", "instrument handle"=w172) -> ("error out"=w162:errorcluster, "instrument handle out"=w164:refnum<k15>)  [unwired: 6 in]
    }
    frame #5 {
      n130 = local read "NI Scope Status"() -> (w176:bool)
      n131 = case shown="True" w176 {
        tunnel: [refnum<k15> refnum ("instrument handle out") w184] -> w178
        tunnel: [errorcluster {"status"=FALSE, "code"=0, "source"=""} ("error out") w183] -> w177
        frame False {
          n132 = Wait (ms)(milliseconds to wait=u32 1) -> ()  [unwired: 1 out]
          n133 = property on="NI Scope Tab" class="TabCtl (strict)"("DisabledEnum"=T3."Disabled and Grayed Out" ("Disabled")) -> ()  [unwired: 2 in, 2 out]
        }
        frame True {
          n134 = stacked-sequence {
            tunnel: [_ w216] -> w184
            tunnel: [_ w215] -> w183
            frame #0 {
              w195 = "\t"
              # "Инициализация файла SEU"
              n135 = local read "Образец №"() -> (w200:string)
              n136 = Build Path(base path="SEU path", name or relative path=w200) -> (appended path=w210:path)
              n137 = Get Date/Time In Seconds() -> (seconds since 1Jan1904=w206:timestamp)
              n138 = call <vilib>:"Check if File or Folder Exists.vi"("path"=w210) -> ("file or folder exists?"=w209:bool, "dup path"=w208:path)  [unwired: 8 in, 1 out]
              n139 = Format Date/Time String(time format string (%c)="SEU %d %m %y %H.%M.%S", seconds (now)=w206) -> (date/time string=w205:string)  [unwired: 1 in]
              n140 = case shown="True" w209 {
                tunnel: w208 -> [w212 w213]
                tunnel: [w211 w213] -> w207
                frame False {
                  n141 = Create Folder(path (use dialog)=w212) -> (created path=w211:path)  [unwired: 2 in, 2 out]
                }
                frame True {
                }
              }
              n142 = Concatenate Strings(w205, ".xls" ("string")) -> (w204:string)
              n143 = Build Path(base path=w207, name or relative path=w204) -> (appended path=w203:path)
              n144 = Open/Create/Replace File(file path (use dialog)=w203, operation (0:open)=T4."open or create", access (0:read/write)=enum16{"read/write", "read-only", "write-only"}."read/write") -> (refnum out=w202:refnum<file>)  [unwired: 3 in, 2 out]
              n145 = property on="NI Scope Tab" class="TabCtl (strict)"("DisabledEnum"=T3."Enabled" ("Disabled")) -> ()  [unwired: 2 in, 2 out]
              n146 = Set File Position(refnum=w202, from (0:start)=enum16{"start", "end", "current"}."end") -> (refnum out=w199:refnum<file>)  [unwired: 2 in, 1 out]
              n147 = Format Into String(initial string=w199, "Time" ("string"), w195, "Voltage, V" ("string"), w195, "Current, A" ("string"), w195, "SEU counter" ("string"), w195, "!!!" ("input 7"), "\r\n") -> (resulting string=→"SEU output file refnum":refnum<file>)  [unwired: 2 in, 1 out]
            }
            frame #1 {
              w221 = 2 items=["None"=1, "Auto Trigger"=2] ("Triggering:Trigger Modifier")
              w219 = u32 0 items=["1 mega ohm"=0, "50 ohms"=2] ("Input Impedance")
              w217 = FALSE  # Reset Device
              n148 = call <instrlib>:"niScope Initialize.vi"("resource name"="NI Scope", "reset device"=w217, "error in"="NI Scope error in") -> ("instrument handle"=w228:refnum<k15>, "error out"=w227:errorcluster)  [unwired: 11 in]
              n149 = call <instrlib>:"niScope Configure Chan Characteristics.vi"("instrument handle"=w228, "channels"="0" ("Channel Name"), "input impedance"=w219, "maximum input frequency"=20000000.0 ("Maximum Input Frequency"), "error in"=w227) -> ("instrument handle out"=w230:refnum<k15>, "error out"=w226:errorcluster)  [unwired: 9 in]
              n150 = call <instrlib>:"niScope Configure Horizontal Timing.vi"("instrument handle"=w230, "enforce realtime"=TRUE ("Enforce Realtime"), "min sample rate"=250000000.0 ("Min Sample Rate"), "reference position"=50.0 ("Reference\nPosition"), "error in"=w226, "min record length"=1000000 ("Min Record Length")) -> ("instrument handle out"=w229:refnum<k15>, "error out"=w215:errorcluster)  [unwired: 8 in]
              n151 = property on="Property Node" class="niScope"(reference=w229, "Trigger Modifier"=w221) -> (reference out=w216:refnum<k15>)  [unwired: 1 in, 1 out]
            }
          }
        }
      }
    }
    frame #6 {
      n152 = local read "NI DMM 1 Status"() -> (w236:bool)
      n153 = local read "NI DMM 2 Status"() -> (w235:bool)
      n154 = case shown="True" w236 {
        tunnel: [refnum<k15> refnum ("instrument handle out") w306] -> w234
        tunnel: [errorcluster {"status"=FALSE, "code"=0, "source"=""} ("error out") w305] -> w233
        frame False {
          n155 = property on="NI DMM 1 Tab" class="TabCtl (strict)"("DisabledEnum"=T3."Disabled and Grayed Out" ("Disabled")) -> ()  [unwired: 2 in, 2 out]
        }
        frame True {
          n156 = local read "NI DMM 1 Option Return"() -> (w308:enum32{"Ampermeter button", "Ohmmeter button"})
          n157 = property on="NI DMM 1 Tab" class="TabCtl (strict)"("DisabledEnum"=T3."Enabled" ("Disabled")) -> ()  [unwired: 2 in, 2 out]
          n158 = stacked-sequence {
            tunnel: w308 -> [w309 _]
            tunnel: [_ w363] -> w306
            tunnel: [_ w362] -> w305
            frame #0 {
              n159 = case shown="\"Ampermeter button\", Default" w309 {
                frame "Ampermeter button", Default {
                  # "Инициализация файла SEU"
                  n160 = local read "Образец №"() -> (w325:string)
                  n161 = Build Path(base path="NI DMM 1 Ampermeter path", name or relative path=w325) -> (appended path=w332:path)
                  n162 = Get Date/Time In Seconds() -> (seconds since 1Jan1904=w328:timestamp)
                  n163 = call <vilib>:"Check if File or Folder Exists.vi"("path"=w332) -> ("file or folder exists?"=w331:bool, "dup path"=w330:path)  [unwired: 8 in, 1 out]
                  n164 = Format Date/Time String(time format string (%c)="NI DMM 1 %d %m %y %H.%M.%S", seconds (now)=w328) -> (date/time string=w327:string)  [unwired: 1 in]
                  n165 = case shown="True" w331 {
                    tunnel: w330 -> [w334 w335]
                    tunnel: [w333 w335] -> w329
                    frame False {
                      n166 = Create Folder(path (use dialog)=w334) -> (created path=w333:path)  [unwired: 2 in, 2 out]
                    }
                    frame True {
                    }
                  }
                  n167 = Concatenate Strings(w327, ".xls" ("string")) -> (w326:string)
                  n168 = Build Path(base path=w329, name or relative path=w326) -> (appended path=w311:path)
                  n169 = Open/Create/Replace File(file path (use dialog)=w311, operation (0:open)=T4."open or create", access (0:read/write)=enum16{"read/write", "read-only", "write-only"}."read/write") -> (refnum out=w322:refnum<file>)  [unwired: 3 in, 2 out]
                  n170 = local write "NI DMM 1 Tab"(enum32{"Ampermeter", "Ohmmeter", "System Panel"}."Ampermeter" ("NI DMM 1 Tab")) -> ()
                  n171 = Set File Position(refnum=w322, from (0:start)=enum16{"start", "end", "current"}."end") -> (refnum out=w314:refnum<file>)  [unwired: 2 in, 1 out]
                  n172 = Format Into String(initial string=w314, "Time" ("string"), "\t", "Current, A" ("string"), "\r\n") -> (resulting string=→"NI DMM 1 Current output file":refnum<file>)  [unwired: 2 in, 1 out]
                }
                frame "Ohmmeter button" {
                  # "Инициализация файла SEU"
                  n173 = local read "Образец №"() -> (w351:string)
                  n174 = Build Path(base path="NI DMM 1 Ohmmeter path", name or relative path=w351) -> (appended path=w358:path)
                  n175 = Get Date/Time In Seconds() -> (seconds since 1Jan1904=w354:timestamp)
                  n176 = call <vilib>:"Check if File or Folder Exists.vi"("path"=w358) -> ("file or folder exists?"=w357:bool, "dup path"=w356:path)  [unwired: 8 in, 1 out]
                  n177 = Format Date/Time String(time format string (%c)="NI DMM 1 %d %m %y %H.%M.%S", seconds (now)=w354) -> (date/time string=w353:string)  [unwired: 1 in]
                  n178 = case shown="True" w357 {
                    tunnel: w356 -> [w360 w361]
                    tunnel: [w359 w361] -> w355
                    frame False {
                      n179 = Create Folder(path (use dialog)=w360) -> (created path=w359:path)  [unwired: 2 in, 2 out]
                    }
                    frame True {
                    }
                  }
                  n180 = Concatenate Strings(w353, ".xls" ("string")) -> (w352:string)
                  n181 = Build Path(base path=w355, name or relative path=w352) -> (appended path=w337:path)
                  n182 = Open/Create/Replace File(file path (use dialog)=w337, operation (0:open)=T4."open or create", access (0:read/write)=enum16{"read/write", "read-only", "write-only"}."read/write") -> (refnum out=w348:refnum<file>)  [unwired: 3 in, 2 out]
                  n183 = local write "NI DMM 1 Tab"(enum32{"Ampermeter", "Ohmmeter", "System Panel"}."Ohmmeter" ("NI DMM 1 Tab")) -> ()
                  n184 = Set File Position(refnum=w348, from (0:start)=enum16{"start", "end", "current"}."end") -> (refnum out=w340:refnum<file>)  [unwired: 2 in, 1 out]
                  n185 = Format Into String(initial string=w340, "Time" ("string"), "\t", "Current, A" ("string"), "\r\n") -> (resulting string=→"NI DMM 1 Resistance output file":refnum<file>)  [unwired: 2 in, 1 out]
                }
              }
            }
            frame #1 {
              n186 = call <instrlib>:"niDMM Initialize.vi"("error in (no error)"="NI DMM 1 error in", "Instrument Descriptor"="NI DMM 1") -> ("error out"=w362:errorcluster, "instrument handle out"=w363:refnum<k15>)  [unwired: 8 in]
            }
          }
        }
      }
      "NI DMM 1 error out" <- w233
      n187 = case shown="True" w235 {
        tunnel: [refnum<k15> refnum ("instrument handle out") w241] -> w237
        tunnel: [errorcluster {"status"=FALSE, "code"=0, "source"=""} ("error out") w242] -> w232
        frame False {
          n188 = property on="NI DMM 2 Tab" class="TabCtl (strict)"("DisabledEnum"=T3."Disabled and Grayed Out" ("Disabled")) -> ()  [unwired: 2 in, 2 out]
        }
        frame True {
          n189 = local read "NI DMM 2 Option Return"() -> (w244:enum32{"Ampermeter button", "Ohmmeter button"})
          n190 = property on="NI DMM 2 Tab" class="TabCtl (strict)"("DisabledEnum"=T3."Enabled" ("Disabled")) -> ()  [unwired: 2 in, 2 out]
          n191 = stacked-sequence {
            tunnel: w244 -> [w245 _]
            tunnel: [_ w299] -> w242
            tunnel: [_ w298] -> w241
            frame #0 {
              n192 = case shown="\"Ohmmeter button\"" w245 {
                frame "Ampermeter button", Default {
                  # "Инициализация файла SEU"
                  n193 = local read "Образец №"() -> (w261:string)
                  n194 = Build Path(base path="NI DMM 2 Ampermeter path", name or relative path=w261) -> (appended path=w268:path)
                  n195 = Get Date/Time In Seconds() -> (seconds since 1Jan1904=w264:timestamp)
                  n196 = call <vilib>:"Check if File or Folder Exists.vi"("path"=w268) -> ("file or folder exists?"=w267:bool, "dup path"=w266:path)  [unwired: 8 in, 1 out]
                  n197 = Format Date/Time String(time format string (%c)="NI DMM 2 %d %m %y %H.%M.%S", seconds (now)=w264) -> (date/time string=w263:string)  [unwired: 1 in]
                  n198 = case shown="True" w267 {
                    tunnel: w266 -> [w270 w271]
                    tunnel: [w269 w271] -> w265
                    frame False {
                      n199 = Create Folder(path (use dialog)=w270) -> (created path=w269:path)  [unwired: 2 in, 2 out]
                    }
                    frame True {
                    }
                  }
                  n200 = Concatenate Strings(w263, ".xls" ("string")) -> (w262:string)
                  n201 = Build Path(base path=w265, name or relative path=w262) -> (appended path=w247:path)
                  n202 = Open/Create/Replace File(file path (use dialog)=w247, operation (0:open)=T4."open or create", access (0:read/write)=enum16{"read/write", "read-only", "write-only"}."read/write") -> (refnum out=w258:refnum<file>)  [unwired: 3 in, 2 out]
                  n203 = Set File Position(refnum=w258, from (0:start)=enum16{"start", "end", "current"}."end") -> (refnum out=w250:refnum<file>)  [unwired: 2 in, 1 out]
                  n204 = Format Into String(initial string=w250, "Time" ("string"), "\t", "Current, A" ("string"), "\r\n") -> (resulting string=→"NI DMM 2 Current output file":refnum<file>)  [unwired: 2 in, 1 out]
                  n205 = local write "NI DMM 2 Tab"(enum32{"Ampermeter", "Ohmmeter", "System Panel"}."Ampermeter" ("NI DMM 2 Tab")) -> ()
                }
                frame "Ohmmeter button" {
                  # "Инициализация файла SEU"
                  n206 = local read "Образец №"() -> (w287:string)
                  n207 = Build Path(base path="NI DMM 2 Ohmmeter path", name or relative path=w287) -> (appended path=w294:path)
                  n208 = Get Date/Time In Seconds() -> (seconds since 1Jan1904=w290:timestamp)
                  n209 = call <vilib>:"Check if File or Folder Exists.vi"("path"=w294) -> ("file or folder exists?"=w293:bool, "dup path"=w292:path)  [unwired: 8 in, 1 out]
                  n210 = Format Date/Time String(time format string (%c)="NI DMM 2 %d %m %y %H.%M.%S", seconds (now)=w290) -> (date/time string=w289:string)  [unwired: 1 in]
                  n211 = case shown="True" w293 {
                    tunnel: w292 -> [w296 w297]
                    tunnel: [w295 w297] -> w291
                    frame False {
                      n212 = Create Folder(path (use dialog)=w296) -> (created path=w295:path)  [unwired: 2 in, 2 out]
                    }
                    frame True {
                    }
                  }
                  n213 = Concatenate Strings(w289, ".xls" ("string")) -> (w288:string)
                  n214 = Build Path(base path=w291, name or relative path=w288) -> (appended path=w273:path)
                  n215 = Open/Create/Replace File(file path (use dialog)=w273, operation (0:open)=T4."open or create", access (0:read/write)=enum16{"read/write", "read-only", "write-only"}."read/write") -> (refnum out=w284:refnum<file>)  [unwired: 3 in, 2 out]
                  n216 = Set File Position(refnum=w284, from (0:start)=enum16{"start", "end", "current"}."end") -> (refnum out=w276:refnum<file>)  [unwired: 2 in, 1 out]
                  n217 = Format Into String(initial string=w276, "Time" ("string"), "\t", "Current, A" ("string"), "\r\n") -> (resulting string=→"NI DMM 2 Resistance output file":refnum<file>)  [unwired: 2 in, 1 out]
                  n218 = local write "NI DMM 2 Tab"(enum32{"Ampermeter", "Ohmmeter", "System Panel"}."Ohmmeter" ("NI DMM 2 Tab")) -> ()
                }
              }
            }
            frame #1 {
              n219 = call <instrlib>:"niDMM Initialize.vi"("error in (no error)"="NI DMM 2 error in", "Instrument Descriptor"="NI DMM 2") -> ("error out"=w299:errorcluster, "instrument handle out"=w298:refnum<k15>)  [unwired: 8 in]
            }
          }
        }
      }
      "NI DMM 2error out" <- w232
    }
    frame #7 {
      n220 = local read "Ophir 1 Status"() -> (w366:bool)
      n221 = case shown="True" w366 {
        frame False {
          n222 = property on="Ophir 1 Tab" class="TabCtl (strict)"("DisabledEnum"=T3."Disabled and Grayed Out" ("Disabled")) -> ()  [unwired: 2 in, 2 out]
        }
        frame True {
          n223 = call "Ophir InitCom.vi"("GPIB Address (default 10)"="Ophir 1 GPIB Address (10)", "Communication (default USB 0)"="Ophir 1 Select Communication Protocol", "USB Channel number (default 0)"="Ophir 1 usb channel", "Port Number (default 2)"="Ophir 1 Port Number (default 2)", "error in (no error)"="Ophir 1 error in (no error)", "Baud Rate (3:9600)"="Ophir 1 Baud Rate (3:9600)") -> ("dup Visa Session"=w374:refnum<visa-resource-name>, "error out"=w373:errorcluster)  [unwired: 1 out]
          n224 = call "Ophir InstrInfo.vi"("Visa Session"=w374, "error in (no error)"=w373) -> ("dup Visa Session"=w387:refnum<visa-resource-name>, "Instrument Info"=w383:string, "error out"=w385:errorcluster)
          n225 = call "Ophir HeadInfo.vi"("Visa Session"=w387, "error in (no error)"=w385) -> ("error out"=w384:errorcluster, "dup Visa Session"=w386:refnum<visa-resource-name>, "Head Info"=w382:string)  [unwired: 6 out]
          n226 = call "Ophir InfoStrings.vi"("error in (no error)"=w384, "Head Info"=w382, "Instrument Info"=w383) -> ("error out"=w381:errorcluster, "Strings Array"=w380:string[])
          n227 = property on="Ophir 1 Info" class="Ring (strict)"("Strings []"=w380) -> ()  [unwired: 2 in, 2 out]
          n228 = property on="Ophir 1 Tab" class="TabCtl (strict)"("DisabledEnum"=T3."Enabled" ("Disabled")) -> ()  [unwired: 2 in, 2 out]
          n229 = call "Ophir ConfigDevice.vi"("Visa Session"=w386, "Measure Choice (0:Power)"=u16 0, "error in (no error)"=w381) -> ("dup Visa Session"=→"Ophir 1 dup Visa Session":refnum<visa-resource-name>, "OK ?"=→"Ophir 1 Initialization":bool, "error out"=→"Ophir 1 error out":errorcluster)  [unwired: 1 out]
        }
      }
    }
    frame #8 {
      n230 = local read "Ophir 2 Status"() -> (w389:bool)
      n231 = case shown="True" w389 {
        frame False {
          n232 = property on="Ophir 2 Tab" class="TabCtl (strict)"("DisabledEnum"=T3."Disabled and Grayed Out" ("Disabled")) -> ()  [unwired: 2 in, 2 out]
        }
        frame True {
          n233 = call "Ophir InitCom.vi"("GPIB Address (default 10)"="Ophir 2 GPIB Address (10)", "Communication (default USB 0)"="Ophir 2 Select Communication Protocol", "USB Channel number (default 0)"="Ophir 2 usb channel", "Port Number (default 2)"="Ophir 2 Port Number (default 2)", "error in (no error)"="Ophir 2 error in (no error)", "Baud Rate (3:9600)"="Ophir 2 Baud Rate (3:9600)") -> ("dup Visa Session"=w397:refnum<visa-resource-name>, "error out"=w396:errorcluster)  [unwired: 1 out]
          n234 = call "Ophir InstrInfo.vi"("Visa Session"=w397, "error in (no error)"=w396) -> ("dup Visa Session"=w410:refnum<visa-resource-name>, "Instrument Info"=w406:string, "error out"=w408:errorcluster)
          n235 = call "Ophir HeadInfo.vi"("Visa Session"=w410, "error in (no error)"=w408) -> ("error out"=w407:errorcluster, "dup Visa Session"=w409:refnum<visa-resource-name>, "Head Info"=w405:string)  [unwired: 6 out]
          n236 = call "Ophir InfoStrings.vi"("error in (no error)"=w407, "Head Info"=w405, "Instrument Info"=w406) -> ("error out"=w404:errorcluster, "Strings Array"=w403:string[])
          n237 = property on="Ophir 2 Info" class="Ring (strict)"("Strings []"=w403) -> ()  [unwired: 2 in, 2 out]
          n238 = property on="Ophir 2 Tab" class="TabCtl (strict)"("DisabledEnum"=T3."Enabled" ("Disabled")) -> ()  [unwired: 2 in, 2 out]
          n239 = call "Ophir ConfigDevice.vi"("Visa Session"=w409, "Measure Choice (0:Power)"=u16 0, "error in (no error)"=w404) -> ("dup Visa Session"=→"Ophir 2 dup Visa Session":refnum<visa-resource-name>, "OK ?"=→"Ophir 2 Initialization":bool, "error out"=→"Ophir 2 error out":errorcluster)  [unwired: 1 out]
        }
      }
    }
    frame #9 {
      w412 = TRUE ("Boolean")
      "Ready Status" <- w412
    }
  }
  n240 = flat-sequence {
    tunnel: [w425] -> w4
    tunnel: w1 -> [w415]
    tunnel: [w452] -> w5
    tunnel: w4 -> [w451]
    tunnel: w2 -> [_]
    tunnel: w5 -> [w502]
    frame #0 {
      w413 = "\t"
      n241 = local read "NI DMM 1 Option Return"() -> (w423:enum32{"Ampermeter button", "Ohmmeter button"})
      n242 = local read "NI DMM 1 Option Return"() -> (w421:enum32{"Ampermeter button", "Ohmmeter button"})
      n243 = Build Path(base path="Full Log Path", name or relative path=w415) -> (appended path=w443:path)
      n244 = Get Date/Time In Seconds() -> (seconds since 1Jan1904=w439:timestamp)
      n245 = case shown="\"Ohmmeter button\"" w423 {
        tunnel: ["DMM 1 Current" ("string") "DMM 2 Resistance" ("string")] -> w422
        frame "Ampermeter button", Default {
        }
        frame "Ohmmeter button" {
        }
      }
      n246 = case shown="\"Ohmmeter button\"" w421 {
        tunnel: ["DMM 1 Current" ("string") "DMM 2 Resistance" ("string")] -> w418
        frame "Ampermeter button", Default {
        }
        frame "Ohmmeter button" {
        }
      }
      n247 = call <vilib>:"Check if File or Folder Exists.vi"("path"=w443) -> ("file or folder exists?"=w442:bool, "dup path"=w441:path)  [unwired: 8 in, 1 out]
      n248 = Format Date/Time String(time format string (%c)="Full Log %d %m %y %H.%M.%S", seconds (now)=w439) -> (date/time string=w438:string)  [unwired: 1 in]
      n249 = case shown="False" w442 {
        tunnel: w441 -> [w449 w450]
        tunnel: [w448 w450] -> w440
        frame False {
          n250 = Create Folder(path (use dialog)=w449) -> (created path=w448:path)  [unwired: 2 in, 2 out]
        }
        frame True {
        }
      }
      n251 = Concatenate Strings(w438, ".xls" ("string")) -> (w437:string)
      n252 = Build Path(base path=w440, name or relative path=w437) -> (appended path=w436:path)
      n253 = Open/Create/Replace File(file path (use dialog)=w436, operation (0:open)=T4."open or create", access (0:read/write)=enum16{"read/write", "read-only", "write-only"}."read/write") -> (refnum out=w435:refnum<file>)  [unwired: 3 in, 2 out]
      n254 = Set File Position(refnum=w435, from (0:start)=enum16{"start", "end", "current"}."end") -> (refnum out=w433:refnum<file>)  [unwired: 2 in, 1 out]
      n255 = Format Into String(initial string=w433, "Time" ("string"), w413, "P1 CH0, V" ("string"), w413, "P1 CH0_cur, A" ("string"), w413, w422, w413, "Ophir 1 Optival Power" ("string"), w413, w413, "P2 CH0, V" ("string"), w413, "P2 CH0_cur, A" ("string"), w413, w418, w413, "Ophir 2 Optival Power" ("string"), "\r\n") -> (resulting string=w425:refnum<file>)  [unwired: 2 in, 1 out]
    }
    frame #1 {
      n256 = while {
        tunnel: [w456] -> w452
        tunnel: w451 -> [w453]
        stop <- w455 stop-if-true
        n257 = local read "P1 CH0 Used"() -> (w459:bool)
        n258 = local read "P2 CH0 Used"() -> (w458:bool)
        n259 = Wait (ms)(milliseconds to wait="Full Log Wait") -> ()  [unwired: 1 out]
        n260 = case shown="True" w459 {
          tunnel: ["" w488] -> w464
          frame False {
          }
          frame True {
            w491 = 6
            w489 = "\t"
            n261 = local read "NI DMM 1 Option Return"() -> (w490:enum32{"Ampermeter button", "Ohmmeter button"})
            n262 = case shown="\"Ohmmeter button\"" w490 {
              tunnel: [w500 w501] -> w496
              frame "Ampermeter button", Default {
                n263 = local read "NI DMM 1 Current"() -> (w500:dbl)
              }
              frame "Ohmmeter button" {
                n264 = local read "NI DMM 1 Resistance"() -> (w501:dbl)
              }
            }
            n265 = local read "P1 CH0, V"() -> (w492:dbl)
            n266 = local read "P1 CH0_cur, A"() -> (w493:dbl)
            n267 = local read "Ophir 1 Real Optical Power"() -> (w498:dbl)
            n268 = Number To Fractional String(number=w492, precision (6)=w491) -> (F-format string=w494:string)  [unwired: 2 in]
            n269 = Number To Fractional String(number=w493, precision (6)=w491) -> (F-format string=w495:string)  [unwired: 2 in]
            n270 = Number To Fractional String(number=w496, precision (6)=w491) -> (F-format string=w497:string)  [unwired: 2 in]
            n271 = Number To Fractional String(number=w498, precision (6)=i16 10) -> (F-format string=w499:string)  [unwired: 2 in]
            n272 = Concatenate Strings(w489, w494, w489, w495, w489, w497, w489, w499, w489) -> (w488:string)
          }
        }
        n273 = case shown="True" w458 {
          tunnel: ["" w473] -> w462
          frame False {
          }
          frame True {
            w482 = 6
            w472 = "\t"
            n274 = local read "NI DMM 2 Option Return"() -> (w483:enum32{"Ampermeter button", "Ohmmeter button"})
            n275 = case shown="\"Ampermeter button\", Default" w483 {
              tunnel: [w484 w485] -> w478
              frame "Ampermeter button", Default {
                n276 = local read "NI DMM 2 Current"() -> (w484:dbl)
              }
              frame "Ohmmeter button" {
                n277 = local read "NI DMM 2 Resistance"() -> (w485:dbl)
              }
            }
            n278 = local read "P2 CH0, V"() -> (w474:dbl)
            n279 = local read "P2 CH0_cur, A"() -> (w481:dbl)
            n280 = local read "Ophir 2 Real Optical Power"() -> (w476:dbl)
            n281 = Number To Fractional String(number=w474, precision (6)=w482) -> (F-format string=w480:string)  [unwired: 2 in]
            n282 = Number To Fractional String(number=w481, precision (6)=w482) -> (F-format string=w479:string)  [unwired: 2 in]
            n283 = Number To Fractional String(number=w478, precision (6)=w482) -> (F-format string=w477:string)  [unwired: 2 in]
            n284 = Number To Fractional String(number=w476, precision (6)=i16 10) -> (F-format string=w475:string)  [unwired: 2 in]
            n285 = Concatenate Strings(w472, w480, w472, w479, w472, w477, w472, w475) -> (w473:string)
          }
        }
        n286 = Or(x=w459, y=w458) -> (x .or. y?=w460:bool)
        n287 = case shown="True" w460 {
          tunnel: ["" ("date/time string") w468] -> w463
          tunnel: ["" "\r\n"] -> w461
          frame False {
          }
          frame True {
            n288 = Format Date/Time String(time format string (%c)="%H:%M:%S:%3u") -> (date/time string=w468:string)  [unwired: 2 in]
          }
        }
        n289 = Concatenate Strings(w463, w464, w462, w461) -> (w457:string)
        n290 = local read "STOP"() -> (w455:bool)
        n291 = Format Into String(initial string=w453, w457) -> (resulting string=w456:refnum<file>)  [unwired: 2 in, 1 out]
      }
    }
    frame #2 {
      n292 = Close File(refnum=w502) -> ()  [unwired: 1 in, 2 out]
    }
  }
  n293 = case shown="True" w8 {
    tunnel: w14 -> [_ w509]
    tunnel: w3 -> [_ _]
    tunnel: w11 -> [_ w506]
    frame False {
    }
    frame True {
      n294 = local read "NI DMM 1 Option Return"() -> (w503:enum32{"Ampermeter button", "Ohmmeter button"})
      n295 = case shown="\"Ampermeter button\", Default" w503 {
        tunnel: w509 -> [w514 w560]
        tunnel: [w513 w559] -> w508
        tunnel: [w512 w558] -> w507
        tunnel: w506 -> [w511 w561]
        tunnel: [w510 w557] -> w505
        frame "Ampermeter button", Default {
          n296 = while {
            tunnel: w514 -> [w526]
            tunnel: [w524] -> w513
            tunnel: [w523] -> w512
            tunnel: w511 -> [w521]
            tunnel: [w517] -> w510
            stop <- w522 stop-if-true
            n297 = flat-sequence {
              tunnel: [w532] -> w527
              tunnel: w526 -> [w530]
              tunnel: w521 -> [w534]
              tunnel: [w531] -> w520
              tunnel: w527 -> [w536]
              tunnel: [w542] -> w525
              tunnel: w520 -> [w541]
              tunnel: [w540] -> w519
              tunnel: [w537] -> w515
              tunnel: w525 -> [w547]
              tunnel: [w548] -> w524
              tunnel: [w547] -> w523
              tunnel: [w546] -> w522
              tunnel: w519 -> [w545]
              tunnel: [w545] -> w518
              tunnel: w515 -> [w544]
              frame #0 {
                w528 = T6 6.5 items=["3 1/2"=3.5, "4 1/2"=4.5, "5 1/2"=5.5, "6 1/2"=6.5, "7 1/2"=7.5] ("Resolution in Digits")
                n298 = Fract/Exp String To Number(string="NI DMM 1 Current Range") -> (number=w533:dbl)  [unwired: 3 in, 1 out]
                n299 = call-poly <instrlib>:"niDMM Config Measurement.vi"("Range"=w533, "Resolution in Digits"=w528, "error in (no error)"=w534, "Function"=niDMM_Function."DC Current" ("Measurement Type"), "instrument handle"=w530) -> ("error out"=w531:errorcluster, "instrument handle out"=w532:refnum<k15>)  [unwired: 5 in]
              }
              frame #1 {
                n300 = call <instrlib>:"niDMM Read.vi"("error in (no error)"=w541, "instrument handle"=w536) -> ("error out"=w540:errorcluster, "Measurement"=w537:dbl, "instrument handle out"=w542:refnum<k15>)  [unwired: 7 in]
                n301 = Fract/Exp String To Number(string="NI DMM 1 units") -> (number=w538:dbl)  [unwired: 3 in, 1 out]
                n302 = Multiply(x=w538, y=w537) -> (x*y=→"NI DMM 1 Current" →"NI DMM 1 Current Char":dbl)
              }
              frame #2 {
                w556 = 6
                n303 = local read "NI DMM 1 Current output file"() -> (w549:refnum<file>)
                n304 = Format Date/Time String(time format string (%c)="%H:%M:%S:%3u") -> (date/time string=w554:string)  [unwired: 2 in]
                n305 = Number To Fractional String(number=w544, width (-)=w556, precision (6)=w556) -> (F-format string=w551:string)  [unwired: 1 in]
                n306 = local read "STOP"() -> (w546:bool)
                n307 = Concatenate Strings(w554, "\t", w551, "\r\n") -> (w552:string)
                n308 = Format Into String(initial string=w549, w552) -> (resulting string=w548:refnum<file>)  [unwired: 2 in, 1 out]
              }
            }
            n309 = Wait (ms)(milliseconds to wait="NI DMM 1 Current Wait") -> ()  [unwired: 1 out]
            n310 = call <vilib>:"Simple Error Handler.vi"("error in (no error)"=w518) -> ("error out"=w517:errorcluster)  [unwired: 1 in, 7 out]
          }
        }
        frame "Ohmmeter button" {
          n311 = while {
            tunnel: w560 -> [w573]
            tunnel: [w571] -> w559
            tunnel: [w570] -> w558
            tunnel: w561 -> [w568]
            tunnel: [w564] -> w557
            stop <- w569 stop-if-true
            n312 = flat-sequence {
              tunnel: [w580] -> w574
              tunnel: w573 -> [w579]
              tunnel: w568 -> [w578]
              tunnel: [w577] -> w567
              tunnel: w574 -> [w590]
              tunnel: [w588] -> w572
              tunnel: w567 -> [w587]
              tunnel: [w586] -> w566
              tunnel: [w583] -> w562
              tunnel: w572 -> [w594]
              tunnel: [w595] -> w571
              tunnel: [w594] -> w570
              tunnel: [w593] -> w569
              tunnel: [w592] -> w565
              tunnel: w566 -> [w592]
              tunnel: w562 -> [w591]
              frame #0 {
                w582 = T6 6.5 items=["3 1/2"=3.5, "4 1/2"=4.5, "5 1/2"=5.5, "6 1/2"=6.5, "7 1/2"=7.5] ("Resolution in Digits")
                n313 = Fract/Exp String To Number(string="NI DMM 1 Resistance Range") -> (number=w575:dbl)  [unwired: 3 in, 1 out]
                n314 = call-poly <instrlib>:"niDMM Config Measurement.vi"("Range"=w575, "Resolution in Digits"=w582, "error in (no error)"=w578, "Function"=niDMM_Function."2-wire Resistance" ("Measurement Type"), "instrument handle"=w579) -> ("error out"=w577:errorcluster, "instrument handle out"=w580:refnum<k15>)  [unwired: 5 in]
              }
              frame #1 {
                n315 = call <instrlib>:"niDMM Read.vi"("error in (no error)"=w587, "instrument handle"=w590) -> ("error out"=w586:errorcluster, "Measurement"=w583:dbl, "instrument handle out"=w588:refnum<k15>)  [unwired: 7 in]
                n316 = Fract/Exp String To Number(string="NI DMM 1 Resistance units") -> (number=w584:dbl)  [unwired: 3 in, 1 out]
                n317 = Multiply(x=w584, y=w583) -> (x*y=→"NI DMM 1 Resistance" →"NI DMM 1 Resistance Char":dbl)
              }
              frame #2 {
                w596 = 6
                n318 = local read "NI DMM 1 Resistance output file"() -> (w603:refnum<file>)
                n319 = Format Date/Time String(time format string (%c)="%H:%M:%S:%3u") -> (date/time string=w598:string)  [unwired: 2 in]
                n320 = Number To Fractional String(number=w591, width (-)=w596, precision (6)=w596) -> (F-format string=w601:string)  [unwired: 1 in]
                n321 = Concatenate Strings(w598, "\t", w601, "\r\n") -> (w600:string)
                n322 = local read "STOP"() -> (w593:bool)
                n323 = Format Into String(initial string=w603, w600) -> (resulting string=w595:refnum<file>)  [unwired: 2 in, 1 out]
              }
            }
            n324 = Wait (ms)(milliseconds to wait="NI DMM 1 Resistance Wait") -> ()  [unwired: 1 out]
            n325 = call <vilib>:"Simple Error Handler.vi"("error in (no error)"=w565) -> ("error out"=w564:errorcluster)  [unwired: 1 in, 7 out]
          }
        }
      }
      n326 = call <instrlib>:"niDMM Close.vi"("error in (no error)"=w505, "instrument handle"=w507) -> ("error out"=w504:errorcluster)  [unwired: 9 in]
      n327 = local write "NI DMM 1 error out"(w504) -> ()
      n328 = Close File(refnum=w508) -> ()  [unwired: 1 in, 2 out]
      n329 = call <vilib>:"Simple Error Handler.vi"("error in (no error)"=w504) -> ()  [unwired: 1 in, 8 out]
    }
  }
  n330 = case shown="True" w7 {
    tunnel: w13 -> [_ w610]
    tunnel: w3 -> [_ _]
    tunnel: w10 -> [_ w607]
    frame False {
    }
    frame True {
      n331 = local read "NI DMM 2 Option Return"() -> (w604:enum32{"Ampermeter button", "Ohmmeter button"})
      n332 = case shown="\"Ampermeter button\", Default" w604 {
        tunnel: w610 -> [w615 w662]
        tunnel: [w614 w660] -> w609
        tunnel: [w613 w659] -> w608
        tunnel: w607 -> [w612 w661]
        tunnel: [w611 w658] -> w606
        frame "Ampermeter button", Default {
          n333 = while {
            tunnel: w615 -> [w627]
            tunnel: [w625] -> w614
            tunnel: [w624] -> w613
            tunnel: w612 -> [w622]
            tunnel: [w618] -> w611
            stop <- w623 stop-if-true
            n334 = flat-sequence {
              tunnel: [w631] -> w628
              tunnel: w627 -> [w629]
              tunnel: w622 -> [w635]
              tunnel: [w630] -> w621
              tunnel: w628 -> [w637]
              tunnel: [w643] -> w626
              tunnel: w621 -> [w642]
              tunnel: [w641] -> w620
              tunnel: [w638] -> w616
              tunnel: w626 -> [w648]
              tunnel: [w649] -> w625
              tunnel: [w648] -> w624
              tunnel: [w647] -> w623
              tunnel: [w646] -> w619
              tunnel: w620 -> [w646]
              tunnel: w616 -> [w645]
              frame #0 {
                w632 = T6 6.5 items=["3 1/2"=3.5, "4 1/2"=4.5, "5 1/2"=5.5, "6 1/2"=6.5, "7 1/2"=7.5] ("Resolution in Digits")
                n335 = Fract/Exp String To Number(string="NI DMM 2 Current Range") -> (number=w634:dbl)  [unwired: 3 in, 1 out]
                n336 = call-poly <instrlib>:"niDMM Config Measurement.vi"("Range"=w634, "Resolution in Digits"=w632, "error in (no error)"=w635, "Function"=niDMM_Function."DC Current" ("Measurement Type"), "instrument handle"=w629) -> ("error out"=w630:errorcluster, "instrument handle out"=w631:refnum<k15>)  [unwired: 5 in]
              }
              frame #1 {
                n337 = call <instrlib>:"niDMM Read.vi"("error in (no error)"=w642, "instrument handle"=w637) -> ("error out"=w641:errorcluster, "Measurement"=w638:dbl, "instrument handle out"=w643:refnum<k15>)  [unwired: 7 in]
                n338 = Fract/Exp String To Number(string="NI DMM 2 units") -> (number=w639:dbl)  [unwired: 3 in, 1 out]
                n339 = Multiply(x=w639, y=w638) -> (x*y=→"NI DMM 2 Current" →"NI DMM 2 Current Char":dbl)
              }
              frame #2 {
                w650 = 6
                n340 = local read "NI DMM 2 Current output file"() -> (w657:refnum<file>)
                n341 = Format Date/Time String(time format string (%c)="%H:%M:%S:%3u") -> (date/time string=w652:string)  [unwired: 2 in]
                n342 = Number To Fractional String(number=w645, width (-)=w650, precision (6)=w650) -> (F-format string=w655:string)  [unwired: 1 in]
                n343 = Concatenate Strings(w652, "\t", w655, "\r\n") -> (w654:string)
                n344 = local read "STOP"() -> (w647:bool)
                n345 = Format Into String(initial string=w657, w654) -> (resulting string=w649:refnum<file>)  [unwired: 2 in, 1 out]
              }
            }
            n346 = Wait (ms)(milliseconds to wait="NI DMM 2 Current Wait") -> ()  [unwired: 1 out]
            n347 = call <vilib>:"Simple Error Handler.vi"("error in (no error)"=w619) -> ("error out"=w618:errorcluster)  [unwired: 1 in, 7 out]
          }
        }
        frame "Ohmmeter button" {
          n348 = while {
            tunnel: w662 -> [w674]
            tunnel: [w672] -> w660
            tunnel: [w671] -> w659
            tunnel: w661 -> [w669]
            tunnel: [w665] -> w658
            stop <- w670 stop-if-true
            n349 = flat-sequence {
              tunnel: [w681] -> w675
              tunnel: w674 -> [w680]
              tunnel: w669 -> [w679]
              tunnel: [w678] -> w668
              tunnel: w675 -> [w686]
              tunnel: [w685] -> w673
              tunnel: w668 -> [w690]
              tunnel: [w689] -> w667
              tunnel: [w684] -> w663
              tunnel: w673 -> [w695]
              tunnel: [w696] -> w672
              tunnel: [w695] -> w671
              tunnel: [w694] -> w670
              tunnel: [w693] -> w666
              tunnel: w667 -> [w693]
              tunnel: w663 -> [w692]
              frame #0 {
                w683 = T6 6.5 items=["3 1/2"=3.5, "4 1/2"=4.5, "5 1/2"=5.5, "6 1/2"=6.5, "7 1/2"=7.5] ("Resolution in Digits")
                n350 = Fract/Exp String To Number(string="NI DMM 2 Resistance Range") -> (number=w677:dbl)  [unwired: 3 in, 1 out]
                n351 = call-poly <instrlib>:"niDMM Config Measurement.vi"("Range"=w677, "Resolution in Digits"=w683, "error in (no error)"=w679, "Function"=niDMM_Function."2-wire Resistance" ("Measurement Type"), "instrument handle"=w680) -> ("error out"=w678:errorcluster, "instrument handle out"=w681:refnum<k15>)  [unwired: 5 in]
              }
              frame #1 {
                n352 = call <instrlib>:"niDMM Read.vi"("error in (no error)"=w690, "instrument handle"=w686) -> ("error out"=w689:errorcluster, "Measurement"=w684:dbl, "instrument handle out"=w685:refnum<k15>)  [unwired: 7 in]
                n353 = Fract/Exp String To Number(string="NI DMM 2 Resistance units") -> (number=w687:dbl)  [unwired: 3 in, 1 out]
                n354 = Multiply(x=w687, y=w684) -> (x*y=→"NI DMM 2 Resistance" →"NI DMM 2 Resistance Char":dbl)
              }
              frame #2 {
                w697 = 6
                n355 = local read "NI DMM 2 Resistance output file"() -> (w704:refnum<file>)
                n356 = Format Date/Time String(time format string (%c)="%H:%M:%S:%3u") -> (date/time string=w699:string)  [unwired: 2 in]
                n357 = Number To Fractional String(number=w692, width (-)=w697, precision (6)=w697) -> (F-format string=w702:string)  [unwired: 1 in]
                n358 = Concatenate Strings(w699, "\t", w702, "\r\n") -> (w701:string)
                n359 = local read "STOP"() -> (w694:bool)
                n360 = Format Into String(initial string=w704, w701) -> (resulting string=w696:refnum<file>)  [unwired: 2 in, 1 out]
              }
            }
            n361 = Wait (ms)(milliseconds to wait="NI DMM 2 Resistance Wait") -> ()  [unwired: 1 out]
            n362 = call <vilib>:"Simple Error Handler.vi"("error in (no error)"=w666) -> ("error out"=w665:errorcluster)  [unwired: 1 in, 7 out]
          }
        }
      }
      n363 = call <instrlib>:"niDMM Close.vi"("error in (no error)"=w606, "instrument handle"=w608) -> ("error out"=w605:errorcluster)  [unwired: 9 in]
      n364 = local write "NI DMM 2error out"(w605) -> ()
      n365 = Close File(refnum=w609) -> ()  [unwired: 1 in, 2 out]
      n366 = call <vilib>:"Simple Error Handler.vi"("error in (no error)"=w605) -> ()  [unwired: 1 in, 8 out]
    }
  }
  n367 = case shown="True" w9 {
    tunnel: w3 -> [_ w710]
    tunnel: w15 -> [_ w706]
    tunnel: w12 -> [_ w705]
    frame False {
    }
    frame True {
      n368 = while {
        tunnel: w706 -> [w737]
        tunnel: [w742] -> w709
        tunnel: [w731] -> w708
        tunnel: [w716] -> w707
        tunnel: w710 -> [_]
        tunnel: w705 -> [w718]
        stop <- w738 stop-if-true
        n369 = flat-sequence {
          tunnel: w737 -> [w750]
          tunnel: [w747] -> w726
          tunnel: w718 -> [w744]
          tunnel: [w743] -> w724
          tunnel: [w757] -> w741
          tunnel: w726 -> [w756]
          tunnel: w724 -> [w753]
          tunnel: [w752] -> w723
          tunnel: [w766] -> w740
          tunnel: w741 -> [w765]
          tunnel: w723 -> [w764]
          tunnel: [w763] -> w722
          tunnel: w740 -> [w770]
          tunnel: [w769] -> w739
          tunnel: w722 -> [w768]
          tunnel: [w767] -> w721
          tunnel: [w787] -> w735
          tunnel: w739 -> [w789]
          tunnel: [w786] -> w733
          tunnel: [w779] -> w729
          tunnel: [w781] -> w728
          tunnel: [w780] -> w727
          tunnel: [w776] -> w725
          tunnel: w721 -> [w775]
          tunnel: [w774] -> w719
          tunnel: w735 -> [w851]
          tunnel: [w851] -> w734
          tunnel: w733 -> [w834]
          tunnel: [w841] -> w732
          tunnel: [w839] -> w730
          tunnel: w729 -> [w838]
          tunnel: w728 -> [w837]
          tunnel: w727 -> [w836]
          tunnel: w725 -> [w832]
          tunnel: [w829] -> w720
          tunnel: w719 -> [w829]
          tunnel: [w857] -> w742
          tunnel: w734 -> [w857]
          tunnel: [w858] -> w738
          tunnel: w732 -> [w856]
          tunnel: [w856] -> w731
          tunnel: w730 -> [_]
          tunnel: w720 -> [w855]
          tunnel: [w855] -> w717
          frame #0 {
            n370 = call <instrlib>:"niScope Configure Vertical.vi"("instrument handle"=w750, "probe attenuation"=1.0 ("Probe Attenuation"), "vertical coupling"="AC/DC/Groun", "channels"="0" ("Channel Name"), "vertical range"="vertical range", "vertical offset"=0.0, "error in"=w744) -> ("instrument handle out"=w747:refnum<k15>, "error out"=w743:errorcluster)  [unwired: 7 in]
          }
          frame #1 {
            w762 = 0 items=["Positive", "Negative"] ("Trigger Slope")
            w761 = u16 1 items=["AC"=0, "DC"=1, "HF Reject"=3, "LF Reject"=4, "AC Plus HF Reject"=1001] ("Coupling")
            n371 = call-poly <instrlib>:"niScope Configure Trigger (poly).vi"("instrument handle"=w756, "trigger window mode"=w762, "trigger coupling"=w761, "trigger source"="Trigger Source", "low level"="Low Level", "high level"="High Level", "error in"=w753, "trigger holdoff"=0.0, "trigger delay"=0.0 ("Trigger Delay")) -> ("instrument handle out"=w757:refnum<k15>, "error out"=w752:errorcluster)  [unwired: 5 in]
          }
          frame #2 {
            n372 = call <instrlib>:"niScope Initiate Acquisition.vi"("instrument handle"=w765, "error in"=w764) -> ("instrument handle out"=w766:refnum<k15>, "error out"=w763:errorcluster)  [unwired: 12 in]
          }
          frame #3 {
            n373 = call-poly <instrlib>:"niScope Fetch (poly).vi"("timeout"=1.0, "error in"=w768, "channels"="0", "instrument handle"=w770) -> ("error out"=w767:errorcluster, "waveform"=→"RealTime Waveform":T1, "instrument handle out"=w769:refnum<k15>)  [unwired: 4 in, 1 out]
          }
          frame #4 {
            # "Во время триггера FALSE"
            n374 = property class="niScope" props=["Auto Triggered", "Trigger Hysteresis"](reference=w789) -> (reference out=w788:refnum<k15>, "Auto Triggered"=w785:bool)  [unwired: 1 in, 2 out]
            n375 = case shown="\"Radio Selection P1 CH0\", Default" "Channel for SEU" {
              tunnel: [w791 w797 w799 w803] -> w781
              tunnel: [w792 w796 w800 w804] -> w780
              tunnel: [w793 w795 w801 w805] -> w779
              tunnel: [w790 w794 w798 w802] -> w777
              frame "Radio Selection P1 CH0", Default {
                n376 = local read "P1 CH0_warning"() -> (w790:bool)
                n377 = local read "P1 CH0_cur, A"() -> (w791:dbl)
                n378 = local read "P1 CH0, V"() -> (w792:dbl)
                n379 = Get Date/Time In Seconds() -> (seconds since 1Jan1904=w793:timestamp)
              }
              frame "Radio Selection P1 CH1" {
                n380 = local read "P1 CH1_warning"() -> (w794:bool)
                n381 = local read "P1CH1_cur, A"() -> (w797:dbl)
                n382 = local read "P1 CH1, V"() -> (w796:dbl)
                n383 = Get Date/Time In Seconds() -> (seconds since 1Jan1904=w795:timestamp)
              }
              frame "Radio Selection P2 CH0" {
                n384 = local read "P2 CH0_warning"() -> (w798:bool)
                n385 = local read "P2 CH0_cur, A"() -> (w799:dbl)
                n386 = local read "P2 CH0, V"() -> (w800:dbl)
                n387 = Get Date/Time In Seconds() -> (seconds since 1Jan1904=w801:timestamp)
              }
              frame "Radio Selection P2 CH1" {
                n388 = local read "P1 CH1_warning"() -> (w802:bool)
                n389 = local read "P2 CH1_cur, A"() -> (w803:dbl)
                n390 = local read "P2 CH1, V"() -> (w804:dbl)
                n391 = Get Date/Time In Seconds() -> (seconds since 1Jan1904=w805:timestamp)
              }
            }
            n392 = Not(x=w785) -> (.not. x?=w784:bool)
            n393 = Not(x=w777) -> (.not. x?=w782:bool)
            n394 = And(x=w782, y=w784) -> (x .and. y?=w783:bool)
            n395 = case shown="True" w783 {
              tunnel: w788 -> [w809 w824]
              tunnel: [w809 w816] -> w787
              tunnel: [FALSE TRUE] -> w786
              tunnel: ["" w813] -> w776
              tunnel: w775 -> [w806 w812]
              tunnel: [w806 w810] -> w774
              frame False {
              }
              frame True {
                w815 = 6
                # "Регистрация SEU"
                n396 = call-poly <instrlib>:"niScope Fetch (poly).vi"("timeout"=1.0, "error in"=w812, "channels"="0", "instrument handle"=w824) -> ("error out"=w811:errorcluster, "waveform"=→"SEU Waveform":T1, "instrument handle out"=w817:refnum<k15>)  [unwired: 4 in, 1 out]
                n397 = call-poly <instrlib>:"niScope Fetch (poly).vi"("timeout"=1.0, "error in"=w811, "numSamples"=1, "channels"="0", "instrument handle"=w817) -> ("error out"=w810:errorcluster, "wfm"=w822:dbl[], "instrument handle out"=w816:refnum<k15>)  [unwired: 3 in, 1 out]
                n398 = Index Array(array=w822, index=0) -> (element=w814:dbl)
                "SEU Last Level" <- w814
                n399 = Number To Fractional String(number=w814, width (-)=w815, precision (6)=w815) -> (F-format string=w813:string)  [unwired: 1 in]
              }
            }
          }
          frame #5 {
            w842 = 6
            w846 = 0
            w845 = 6
            w833 = "\t"
            # "Регистрация SEU"
            n400 = case shown="True" w834 {
              tunnel: [w852 w853] -> w835
              frame False {
                n401 = local read "SEU_Counter"() -> (w852:u32)
              }
              frame True {
                n402 = local read "SEU_Counter"() -> (w854:u32)
                n403 = Increment(x=w854) -> (x+1=w853:u32)
                "SEU_Counter" <- w853
              }
            }
            n404 = Format Date/Time String(time format string (%c)="%H:%M:%S:%3u", seconds (now)=w838) -> (date/time string=w848:string)  [unwired: 1 in]
            n405 = local read "SEU output file refnum"() -> (w828:refnum<file>)
            n406 = Number To Fractional String(number=w836, width (-)=w842, precision (6)=w842) -> (F-format string=w847:string)  [unwired: 1 in]
            n407 = Number To Fractional String(number=w837, width (-)=w845, precision (6)=w845) -> (F-format string=w849:string)  [unwired: 1 in]
            n408 = Number To Fractional String(number=w835, width (-)=w846, precision (6)=w846) -> (F-format string=w850:string)  [unwired: 1 in]
            n409 = Select(t="???", s=w834, f="") -> (s? t:f=w831:string)
            n410 = Concatenate Strings(w848, w833, w847, w833, w849, w833, w850, w833, w832, w833, w831, "\r\n") -> (w839:string)
            n411 = Format Into String(initial string=w828, w839) -> (resulting string=w841:refnum<file>)  [unwired: 2 in, 1 out]
            "SEU_warning" <- w834
            "SEU" <- w834
          }
          frame #6 {
            n412 = local read "STOP"() -> (w858:bool)
          }
        }
        n413 = Wait (ms)(milliseconds to wait=u32 1) -> ()  [unwired: 1 out]
        n414 = call <vilib>:"Simple Error Handler.vi"("error in (no error)"=w717) -> ("error out"=w716:errorcluster)  [unwired: 1 in, 7 out]
        "NI Scope error out" <- w716
      }
      n415 = flat-sequence {
        tunnel: w709 -> [w715]
        tunnel: w708 -> [w714]
        tunnel: w707 -> [w713]
        frame #0 {
          n416 = Close File(refnum=w714) -> ()  [unwired: 1 in, 2 out]
          n417 = call <instrlib>:"niScope Close.vi"("instrument handle"=w715, "error in"=w713) -> ("error out"=w712:errorcluster)  [unwired: 13 in]
          n418 = call <vilib>:"Simple Error Handler.vi"("error in (no error)"=w712) -> ("error out"=w711:errorcluster)  [unwired: 1 in, 7 out]
          n419 = local write "NI Scope error out"(w711) -> ()
        }
      }
    }
  }
  n420 = while {
    tunnel: w23 -> [w870]
    tunnel: [w869] -> _
    tunnel: w22 -> [w867]
    tunnel: [w866] -> w25
    tunnel: [w865] -> w24
    tunnel: [w861] -> w20
    tunnel: [w859] -> w19
    tunnel: w18 -> [w864]
    tunnel: w17 -> [w863]
    tunnel: w16 -> [_]
    stop <- w869 stop-if-true
    # "Инициализация источников"
    n421 = Wait (ms)(milliseconds to wait=u32 1) -> ()  [unwired: 1 out]
    n422 = flat-sequence {
      tunnel: w870 -> [w946]
      tunnel: [w921] -> w869
      tunnel: w867 -> [w879]
      tunnel: [w878] -> w866
      tunnel: [w877] -> w865
      tunnel: [w876] -> w862
      tunnel: [w875] -> w860
      tunnel: w864 -> [w874]
      tunnel: w863 -> [w871]
      frame #0 {
        w880 = T7 0 items=["Current", "Voltage"] ("measurement type")
        n423 = local read "Power OFF"() -> (w898:bool)
        n424 = call <instrlib>:"niDCPower Configure Current Limit.vi"("error in (no error)"=w874, "current limit"="P1 CH0_curlim, A", "channel name"="0", "instrument handle"=w946) -> ("error out"=w873:errorcluster, "instrument handle out"=w935:refnum<k15>)  [unwired: 6 in]
        n425 = call <instrlib>:"niDCPower Configure Current Limit.vi"("current limit"="P1 CH1_curlim, A", "channel name"="1", "instrument handle"=w946) -> ("instrument handle out"=w932:refnum<k15>)  [unwired: 7 in, 1 out]
        n426 = call <instrlib>:"niDCPower Configure Current Limit.vi"("error in (no error)"=w871, "current limit"="P2 CH0_curlim, A", "channel name"="0", "instrument handle"=w879) -> ("error out"=w872:errorcluster, "instrument handle out"=w911:refnum<k15>)  [unwired: 6 in]
        n427 = call <instrlib>:"niDCPower Configure Current Limit.vi"("current limit"="P2 CH1_curlim, A", "channel name"="1", "instrument handle"=w879) -> ("instrument handle out"=w890:refnum<k15>)  [unwired: 7 in, 1 out]
        n428 = local read "Power OFF"() -> (w920:bool)
        n429 = local read "Power OFF"() -> (w883:bool)
        n430 = local read "Power OFF"() -> (w903:bool)
        n431 = call <instrlib>:"niDCPower Configure Voltage Level.vi"("error in (no error)"=w873, "voltage level"="P1 CH0, V", "channel name"="0", "instrument handle"=w935) -> ("error out"=w940:errorcluster, "instrument handle out"=w941:refnum<k15>)  [unwired: 6 in]
        n432 = call <instrlib>:"niDCPower Configure Voltage Level.vi"("voltage level"="P1 CH1, V", "channel name"="1", "instrument handle"=w932) -> ("error out"=w938:errorcluster, "instrument handle out"=w939:refnum<k15>)  [unwired: 7 in]
        n433 = call <instrlib>:"niDCPower Configure Voltage Level.vi"("error in (no error)"=w872, "voltage level"="P2 CH0, V", "channel name"="0", "instrument handle"=w911) -> ("error out"=w908:errorcluster, "instrument handle out"=w907:refnum<k15>)  [unwired: 6 in]
        n434 = call <instrlib>:"niDCPower Configure Voltage Level.vi"("voltage level"="P2 CH1, V", "channel name"="1", "instrument handle"=w890) -> ("error out"=w893:errorcluster, "instrument handle out"=w894:refnum<k15>)  [unwired: 7 in]
        n435 = Select(t=FALSE, s=w898, f="P1 CH0") -> (s? t:f=w897:bool)
        n436 = Select(t=FALSE, s=w920, f="P1 CH1") -> (s? t:f=w917:bool)
        n437 = Select(t=FALSE, s=w883, f="P2 CH1") -> (s? t:f=w881:bool)
        n438 = Select(t=FALSE, s=w903, f="P2 CH0") -> (s? t:f=w902:bool)
        n439 = call <instrlib>:"niDCPower Configure Output Enabled.vi"("error in (no error)"=w940, "output enabled"=w897, "channel name"="0", "instrument handle"=w941) -> ("error out"=w943:errorcluster, "instrument handle out"=w942:refnum<k15>)  [unwired: 6 in]
        n440 = call <instrlib>:"niDCPower Configure Output Enabled.vi"("error in (no error)"=w938, "output enabled"=w917, "channel name"="1", "instrument handle"=w939) -> ("error out"=w945:errorcluster, "instrument handle out"=w944:refnum<k15>)  [unwired: 6 in]
        n441 = call <instrlib>:"niDCPower Configure Output Enabled.vi"("error in (no error)"=w908, "output enabled"=w902, "channel name"="0", "instrument handle"=w907) -> ("error out"=w905:errorcluster, "instrument handle out"=w906:refnum<k15>)  [unwired: 6 in]
        n442 = call <instrlib>:"niDCPower Configure Output Enabled.vi"("error in (no error)"=w893, "output enabled"=w881, "channel name"="1", "instrument handle"=w894) -> ("error out"=w896:errorcluster, "instrument handle out"=w895:refnum<k15>)  [unwired: 6 in]
        n443 = call <instrlib>:"niDCPower Measure.vi"("error in (no error)"=w943, "measurement type"=w880, "channel name"="0", "instrument handle"=w942) -> ("error out"=w876:errorcluster, "measurement"=→"P1 CH0_cur, A" →"P1 CH0_char":dbl, "instrument handle out"=w878:refnum<k15>)  [unwired: 5 in]
        n444 = call <instrlib>:"niDCPower Measure.vi"("error in (no error)"=w945, "measurement type"=w880, "channel name"="1", "instrument handle"=w944) -> ("measurement"=→"P1CH1_cur, A" →"P1 CH1_char":dbl)  [unwired: 5 in, 2 out]
        n445 = call <instrlib>:"niDCPower Measure.vi"("error in (no error)"=w905, "measurement type"=w880, "channel name"="0", "instrument handle"=w906) -> ("error out"=w875:errorcluster, "measurement"=→"P2 CH0_cur, A" →"P2 CH0_char":dbl, "instrument handle out"=w877:refnum<k15>)  [unwired: 5 in]
        n446 = call <instrlib>:"niDCPower Measure.vi"("error in (no error)"=w896, "measurement type"=w880, "channel name"="1", "instrument handle"=w895) -> ("measurement"=→"P2 CH1_cur, A" →"P2 CH1_char":dbl)  [unwired: 5 in, 2 out]
        n447 = local read "Power OFF"() -> (w921:bool)
      }
    }
    n448 = call <vilib>:"Simple Error Handler.vi"("error in (no error)"=w860) -> ("error out"=w859:errorcluster)  [unwired: 1 in, 7 out]
    "DC Power 2 error out" <- w859
    n449 = call <vilib>:"Simple Error Handler.vi"("error in (no error)"=w862) -> ("error out"=w861:errorcluster)  [unwired: 1 in, 7 out]
    "DC Power 1 error out" <- w861
  }
  n450 = while {
    tunnel: w3 -> [_]
    stop <- w960 stop-if-true
    n451 = Wait (ms)(milliseconds to wait=u32 100) -> ()  [unwired: 1 out]
    n452 = local read "STOP"() -> (w950:bool)
    n453 = local read "STOP"() -> (w947:bool)
    n454 = Or(x="P1 CH0 Used", y=w950) -> (x .or. y?=w952:bool)
    n455 = Or(x="P1 CH1 Used", y=w947) -> (x .or. y?=w949:bool)
    n456 = case shown="True" w952 {
      frame False {
        n457 = property on="P1 CH0" class="Bool (strict)"("DisabledEnum"=T3."Disabled and Grayed Out" ("Disabled")) -> ()  [unwired: 2 in, 2 out]
        n458 = property on="P1 CH0_char" class="WFChart (strict)"("DisabledEnum"=T3."Disabled and Grayed Out" ("Disabled")) -> ()  [unwired: 2 in, 2 out]
        n459 = property on="P1 CH0, V" class="DigNum (strict)"("DisabledEnum"=T3."Disabled and Grayed Out" ("Disabled")) -> ()  [unwired: 2 in, 2 out]
        n460 = property on="P1 CH0_curlim, A" class="DigNum (strict)"("DisabledEnum"=T3."Disabled and Grayed Out" ("Disabled")) -> ()  [unwired: 2 in, 2 out]
        n461 = property on="P1 CH0_cur, A" class="DigNum (strict)"("DisabledEnum"=T3."Disabled and Grayed Out" ("Disabled")) -> ()  [unwired: 2 in, 2 out]
        n462 = property on="P1 CH0_selcur, A" class="DigNum (strict)"("DisabledEnum"=T3."Disabled and Grayed Out" ("Disabled")) -> ()  [unwired: 2 in, 2 out]
        n463 = property on="P1 CH0_counter" class="DigNum (strict)"("DisabledEnum"=T3."Disabled and Grayed Out" ("Disabled")) -> ()  [unwired: 2 in, 2 out]
        n464 = property on="P1 CH0_warning" class="Bool (strict)"("DisabledEnum"=T3."Disabled and Grayed Out" ("Disabled")) -> ()  [unwired: 2 in, 2 out]
      }
      frame True {
        n465 = property on="P1 CH0" class="Bool (strict)"("DisabledEnum"=T3."Enabled" ("Disabled")) -> ()  [unwired: 2 in, 2 out]
        n466 = property on="P1 CH0_char" class="WFChart (strict)"("DisabledEnum"=T3."Enabled" ("Disabled")) -> ()  [unwired: 2 in, 2 out]
        n467 = property on="P1 CH0, V" class="DigNum (strict)"("DisabledEnum"=T3."Enabled" ("Disabled")) -> ()  [unwired: 2 in, 2 out]
        n468 = property on="P1 CH0_curlim, A" class="DigNum (strict)"("DisabledEnum"=T3."Enabled" ("Disabled")) -> ()  [unwired: 2 in, 2 out]
        n469 = property on="P1 CH0_cur, A" class="DigNum (strict)"("DisabledEnum"=T3."Enabled" ("Disabled")) -> ()  [unwired: 2 in, 2 out]
        n470 = property on="P1 CH0_selcur, A" class="DigNum (strict)"("DisabledEnum"=T3."Enabled" ("Disabled")) -> ()  [unwired: 2 in, 2 out]
        n471 = property on="P1 CH0_counter" class="DigNum (strict)"("DisabledEnum"=T3."Enabled" ("Disabled")) -> ()  [unwired: 2 in, 2 out]
        n472 = property on="P1 CH0_warning" class="Bool (strict)"("DisabledEnum"=T3."Enabled" ("Disabled")) -> ()  [unwired: 2 in, 2 out]
      }
    }
    n473 = case shown="False" w949 {
      frame False {
        n474 = property on="P1 CH1" class="Bool (strict)"("DisabledEnum"=T3."Disabled and Grayed Out" ("Disabled")) -> ()  [unwired: 2 in, 2 out]
        n475 = property on="P1 CH1_char" class="WFChart (strict)"("DisabledEnum"=T3."Disabled and Grayed Out" ("Disabled")) -> ()  [unwired: 2 in, 2 out]
        n476 = property on="P1 CH1, V" class="DigNum (strict)"("DisabledEnum"=T3."Disabled and Grayed Out" ("Disabled")) -> ()  [unwired: 2 in, 2 out]
        n477 = property on="P1 CH1_curlim, A" class="DigNum (strict)"("DisabledEnum"=T3."Disabled and Grayed Out" ("Disabled")) -> ()  [unwired: 2 in, 2 out]
        n478 = property on="P1CH1_cur, A" class="DigNum (strict)"("DisabledEnum"=T3."Disabled and Grayed Out" ("Disabled")) -> ()  [unwired: 2 in, 2 out]
        n479 = property on="P1 CH1_selcur, A" class="DigNum (strict)"("DisabledEnum"=T3."Disabled and Grayed Out" ("Disabled")) -> ()  [unwired: 2 in, 2 out]
        n480 = property on="P1 CH1_counter" class="DigNum (strict)"("DisabledEnum"=T3."Disabled and Grayed Out" ("Disabled")) -> ()  [unwired: 2 in, 2 out]
        n481 = property on="P1 CH1_warning" class="Bool (strict)"("DisabledEnum"=T3."Disabled and Grayed Out" ("Disabled")) -> ()  [unwired: 2 in, 2 out]
      }
      frame True {
        n482 = property on="P1 CH1" class="Bool (strict)"("DisabledEnum"=T3."Enabled" ("Disabled")) -> ()  [unwired: 2 in, 2 out]
        n483 = property on="P1 CH1_char" class="WFChart (strict)"("DisabledEnum"=T3."Enabled" ("Disabled")) -> ()  [unwired: 2 in, 2 out]
        n484 = property on="P1 CH1, V" class="DigNum (strict)"("DisabledEnum"=T3."Enabled" ("Disabled")) -> ()  [unwired: 2 in, 2 out]
        n485 = property on="P1 CH1_curlim, A" class="DigNum (strict)"("DisabledEnum"=T3."Enabled" ("Disabled")) -> ()  [unwired: 2 in, 2 out]
        n486 = property on="P1CH1_cur, A" class="DigNum (strict)"("DisabledEnum"=T3."Enabled" ("Disabled")) -> ()  [unwired: 2 in, 2 out]
        n487 = property on="P1 CH1_selcur, A" class="DigNum (strict)"("DisabledEnum"=T3."Enabled" ("Disabled")) -> ()  [unwired: 2 in, 2 out]
        n488 = property on="P1 CH1_counter" class="DigNum (strict)"("DisabledEnum"=T3."Enabled" ("Disabled")) -> ()  [unwired: 2 in, 2 out]
        n489 = property on="P1 CH1_warning" class="Bool (strict)"("DisabledEnum"=T3."Enabled" ("Disabled")) -> ()  [unwired: 2 in, 2 out]
      }
    }
    n490 = local read "STOP"() -> (w956:bool)
    n491 = local read "STOP"() -> (w953:bool)
    n492 = Or(x="P2 CH0 Used", y=w953) -> (x .or. y?=w955:bool)
    n493 = Or(x="P2 CH1 Used", y=w956) -> (x .or. y?=w957:bool)
    n494 = case shown="True" w955 {
      frame False {
        n495 = property on="P2 CH0" class="Bool (strict)"("DisabledEnum"=T3."Disabled and Grayed Out" ("Disabled")) -> ()  [unwired: 2 in, 2 out]
        n496 = property on="P2 CH0_char" class="WFChart (strict)"("DisabledEnum"=T3."Disabled and Grayed Out" ("Disabled")) -> ()  [unwired: 2 in, 2 out]
        n497 = property on="P2 CH0, V" class="DigNum (strict)"("DisabledEnum"=T3."Disabled and Grayed Out" ("Disabled")) -> ()  [unwired: 2 in, 2 out]
        n498 = property on="P2 CH0_curlim, A" class="DigNum (strict)"("DisabledEnum"=T3."Disabled and Grayed Out" ("Disabled")) -> ()  [unwired: 2 in, 2 out]
        n499 = property on="P2 CH0_cur, A" class="DigNum (strict)"("DisabledEnum"=T3."Disabled and Grayed Out" ("Disabled")) -> ()  [unwired: 2 in, 2 out]
        n500 = property on="P2 CH0_selcur, A" class="DigNum (strict)"("DisabledEnum"=T3."Disabled and Grayed Out" ("Disabled")) -> ()  [unwired: 2 in, 2 out]
        n501 = property on="P2 CH0_counter" class="DigNum (strict)"("DisabledEnum"=T3."Disabled and Grayed Out" ("Disabled")) -> ()  [unwired: 2 in, 2 out]
        n502 = property on="P2 CH0_warning" class="Bool (strict)"("DisabledEnum"=T3."Disabled and Grayed Out" ("Disabled")) -> ()  [unwired: 2 in, 2 out]
      }
      frame True {
        n503 = property on="P2 CH0" class="Bool (strict)"("DisabledEnum"=T3."Enabled" ("Disabled")) -> ()  [unwired: 2 in, 2 out]
        n504 = property on="P2 CH0_char" class="WFChart (strict)"("DisabledEnum"=T3."Enabled" ("Disabled")) -> ()  [unwired: 2 in, 2 out]
        n505 = property on="P2 CH0, V" class="DigNum (strict)"("DisabledEnum"=T3."Enabled" ("Disabled")) -> ()  [unwired: 2 in, 2 out]
        n506 = property on="P2 CH0_curlim, A" class="DigNum (strict)"("DisabledEnum"=T3."Enabled" ("Disabled")) -> ()  [unwired: 2 in, 2 out]
        n507 = property on="P2 CH0_cur, A" class="DigNum (strict)"("DisabledEnum"=T3."Enabled" ("Disabled")) -> ()  [unwired: 2 in, 2 out]
        n508 = property on="P2 CH0_selcur, A" class="DigNum (strict)"("DisabledEnum"=T3."Enabled" ("Disabled")) -> ()  [unwired: 2 in, 2 out]
        n509 = property on="P2 CH0_counter" class="DigNum (strict)"("DisabledEnum"=T3."Enabled" ("Disabled")) -> ()  [unwired: 2 in, 2 out]
        n510 = property on="P2 CH0_warning" class="Bool (strict)"("DisabledEnum"=T3."Enabled" ("Disabled")) -> ()  [unwired: 2 in, 2 out]
      }
    }
    n511 = case shown="True" w957 {
      frame False {
        n512 = property on="P2 CH1" class="Bool (strict)"("DisabledEnum"=T3."Disabled and Grayed Out" ("Disabled")) -> ()  [unwired: 2 in, 2 out]
        n513 = property on="P2 CH1_char" class="WFChart (strict)"("DisabledEnum"=T3."Disabled and Grayed Out" ("Disabled")) -> ()  [unwired: 2 in, 2 out]
        n514 = property on="P2 CH1, V" class="DigNum (strict)"("DisabledEnum"=T3."Disabled and Grayed Out" ("Disabled")) -> ()  [unwired: 2 in, 2 out]
        n515 = property on="P2 CH1_curlim, A" class="DigNum (strict)"("DisabledEnum"=T3."Disabled and Grayed Out" ("Disabled")) -> ()  [unwired: 2 in, 2 out]
        n516 = property on="P2 CH1_cur, A" class="DigNum (strict)"("DisabledEnum"=T3."Disabled and Grayed Out" ("Disabled")) -> ()  [unwired: 2 in, 2 out]
        n517 = property on="P2 CH1_selcur, A" class="DigNum (strict)"("DisabledEnum"=T3."Disabled and Grayed Out" ("Disabled")) -> ()  [unwired: 2 in, 2 out]
        n518 = property on="P2 CH1_counter" class="DigNum (strict)"("DisabledEnum"=T3."Disabled and Grayed Out" ("Disabled")) -> ()  [unwired: 2 in, 2 out]
        n519 = property on="P2 CH1_warning" class="Bool (strict)"("DisabledEnum"=T3."Disabled and Grayed Out" ("Disabled")) -> ()  [unwired: 2 in, 2 out]
      }
      frame True {
        n520 = property on="P2 CH1" class="Bool (strict)"("DisabledEnum"=T3."Enabled" ("Disabled")) -> ()  [unwired: 2 in, 2 out]
        n521 = property on="P2 CH1_char" class="WFChart (strict)"("DisabledEnum"=T3."Enabled" ("Disabled")) -> ()  [unwired: 2 in, 2 out]
        n522 = property on="P2 CH1, V" class="DigNum (strict)"("DisabledEnum"=T3."Enabled" ("Disabled")) -> ()  [unwired: 2 in, 2 out]
        n523 = property on="P2 CH1_curlim, A" class="DigNum (strict)"("DisabledEnum"=T3."Enabled" ("Disabled")) -> ()  [unwired: 2 in, 2 out]
        n524 = property on="P2 CH1_cur, A" class="DigNum (strict)"("DisabledEnum"=T3."Enabled" ("Disabled")) -> ()  [unwired: 2 in, 2 out]
        n525 = property on="P2 CH1_selcur, A" class="DigNum (strict)"("DisabledEnum"=T3."Enabled" ("Disabled")) -> ()  [unwired: 2 in, 2 out]
        n526 = property on="P2 CH1_counter" class="DigNum (strict)"("DisabledEnum"=T3."Enabled" ("Disabled")) -> ()  [unwired: 2 in, 2 out]
        n527 = property on="P2 CH1_warning" class="Bool (strict)"("DisabledEnum"=T3."Enabled" ("Disabled")) -> ()  [unwired: 2 in, 2 out]
      }
    }
    n528 = local read "STOP"() -> (w960:bool)
  }
  n529 = while {
    shift-right: [w1036] -> _
    shift-left: FALSE -> [w1042]
    shift-right: [w1035] -> _
    shift-left: FALSE -> [w1041]
    shift-right: [w1037] -> _
    shift-left: FALSE -> [w1040]
    shift-right: [w1038] -> _
    shift-left: FALSE -> [w1039]
    shift-right: [w1031] -> _
    shift-left: FALSE -> [w1032]
    shift-right: [w1029] -> _
    shift-left: FALSE -> [w1030]
    shift-right: [w1027] -> _
    shift-left: FALSE -> [w1028]
    shift-right: [w1025] -> _
    shift-left: FALSE -> [w1026]
    tunnel: w3 -> [_]
    stop <- w1033 stop-if-true
    # "Включение / выключение образцов"
    n530 = stacked-sequence {
      tunnel: w1042 -> [w1086 _]
      tunnel: [w1082 _] -> w1036
      tunnel: w1041 -> [w1078 _]
      tunnel: [w1077 _] -> w1035
      tunnel: w1040 -> [w1076 _]
      tunnel: w1039 -> [w1070 _]
      tunnel: [w1068 _] -> w1038
      tunnel: [w1067 _] -> w1037
      tunnel: [_ w1103] -> w1033
      tunnel: w1032 -> [w1064 _]
      tunnel: [w1061 _] -> w1031
      tunnel: w1030 -> [w1060 _]
      tunnel: [w1055 _] -> w1029
      tunnel: w1028 -> [w1050 _]
      tunnel: [w1049 _] -> w1027
      tunnel: w1026 -> [w1044 _]
      tunnel: [w1045 _] -> w1025
      frame #0 {
        n531 = local read "P1 CH0 Used"() -> (w1061:bool)
        n532 = local read "P1 CH1 Used"() -> (w1055:bool)
        n533 = local read "P2 CH0 Used"() -> (w1049:bool)
        n534 = local read "P2 CH1 Used"() -> (w1045:bool)
        n535 = local read "P1 CH1"() -> (w1067:bool)
        n536 = local read "P2 CH1"() -> (w1082:bool)
        n537 = local read "P2 CH0"() -> (w1077:bool)
        n538 = local read "P1 CH0"() -> (w1068:bool)
        n539 = local read "STOP"() -> (w1057:bool)
        n540 = local read "STOP"() -> (w1052:bool)
        n541 = local read "STOP"() -> (w1065:bool)
        n542 = Less?(x=w1067, y=w1076) -> (x < y?=w1058:bool)
        n543 = Less?(x=w1082, y=w1086) -> (x < y?=w1048:bool)
        n544 = Less?(x=w1077, y=w1078) -> (x < y?=w1054:bool)
        n545 = Less?(x=w1049, y=w1050) -> (x < y?=w1051:bool)
        n546 = Less?(x=w1068, y=w1070) -> (x < y?=w1066:bool)
        n547 = Not(x=w1057) -> (.not. x?=w1075:bool)
        n548 = Greater?(x=w1067, y=w1076) -> (0:w1074:bool)
        n549 = Not(x="STOP") -> (.not. x?=w1084:bool)
        n550 = Not(x=w1052) -> (.not. x?=w1080:bool)
        n551 = Greater?(x=w1082, y=w1086) -> (0:w1083:bool)
        n552 = Not(x=w1065) -> (.not. x?=w1071:bool)
        n553 = Greater?(x=w1077, y=w1078) -> (0:w1081:bool)
        n554 = Greater?(x=w1068, y=w1070) -> (0:w1072:bool)
        n555 = Less?(x=w1045, y=w1044) -> (x < y?=w1043:bool)
        n556 = Less?(x=w1061, y=w1064) -> (x < y?=w1063:bool)
        n557 = Less?(x=w1055, y=w1060) -> (x < y?=w1056:bool)
        n558 = And(x=w1075, y=w1074) -> (x .and. y?=w1073:bool)
        n559 = Compound Arithmetic op=OR(w1054, w1052, w1051) -> (w1053:bool)
        n560 = And(x=w1084, y=w1083) -> (x .and. y?=w1085:bool)
        n561 = And(x=w1080, y=w1081) -> (x .and. y?=w1079:bool)
        n562 = Compound Arithmetic op=OR(w1048, "STOP", w1043) -> (w1046:bool)
        n563 = And(x=w1071, y=w1072) -> (x .and. y?=w1069:bool)
        n564 = Compound Arithmetic op=OR(w1066, w1065, w1063) -> (w1062:bool)
        n565 = Compound Arithmetic op=OR(w1058, w1057, w1056) -> (w1059:bool)
        n566 = stacked-sequence {
          tunnel: w1069 -> [w1092]
          tunnel: w1062 -> [w1091]
          frame #0 {
            n567 = case shown="True" w1092 {
              frame False {
              }
              frame True {
                # "ON"
                n568 = local write "P1 CH0"(TRUE ("P1 CH0")) -> ()
              }
            }
            n569 = case shown="True" w1091 {
              frame False {
              }
              frame True {
                # "OFF"
                n570 = local write "P1 CH0"(FALSE ("P1 CH0")) -> ()
              }
            }
          }
        }
        n571 = stacked-sequence {
          tunnel: w1073 -> [w1088]
          tunnel: w1059 -> [w1087]
          frame #0 {
            n572 = case shown="True" w1088 {
              frame False {
              }
              frame True {
                # "ON"
                n573 = local write "P1 CH1"(TRUE ("P1 CH1")) -> ()
              }
            }
            n574 = case shown="True" w1087 {
              frame False {
              }
              frame True {
                # "OFF"
                n575 = local write "P1 CH1"(FALSE ("P1 CH0")) -> ()
              }
            }
          }
        }
        n576 = stacked-sequence {
          tunnel: w1079 -> [w1096]
          tunnel: w1053 -> [w1095]
          frame #0 {
            n577 = case shown="True" w1096 {
              frame False {
              }
              frame True {
                # "ON"
                n578 = local write "P2 CH0"(TRUE ("P2 CH0")) -> ()
              }
            }
            n579 = case shown="True" w1095 {
              frame False {
              }
              frame True {
                # "OFF"
                n580 = local write "P2 CH0"(FALSE ("P1 CH0")) -> ()
              }
            }
          }
        }
        n581 = stacked-sequence {
          tunnel: w1085 -> [w1100]
          tunnel: w1046 -> [w1099]
          frame #0 {
            n582 = case shown="True" w1100 {
              frame False {
              }
              frame True {
                # "ON"
                n583 = local write "P2 CH1"(TRUE ("P2 CH1")) -> ()
              }
            }
            n584 = case shown="True" w1099 {
              frame False {
              }
              frame True {
                # "OFF"
                n585 = local write "P2 CH1"(FALSE ("P1 CH0")) -> ()
              }
            }
          }
        }
      }
      frame #1 {
        n586 = local read "STOP"() -> (w1103:bool)
      }
    }
    "Power OFF" <- w1033
    n587 = Wait (ms)(milliseconds to wait=u32 1) -> ()  [unwired: 1 out]
  }
  n588 = while {
    shift-right: [w1112] -> _
    shift-left: FALSE -> [w1114]
    tunnel: [w1104] -> _
    tunnel: [w1113] -> w30
    shift-right: [w1110] -> _
    shift-left: FALSE -> [w1111]
    shift-right: [w1108] -> _
    shift-left: FALSE -> [w1109]
    shift-right: [w1107] -> _
    shift-left: FALSE -> [w1106]
    tunnel: [w1104] -> w21
    tunnel: w3 -> [_]
    tunnel: w3 -> [_]
    tunnel: w3 -> [_]
    stop <- w1104 stop-if-true
    n589 = Wait (ms)(milliseconds to wait="SEL Time Cycle") -> ()  [unwired: 1 out]
    n590 = stacked-sequence {
      seq-local: [w1118 _ _ _] -> [_ _ w1283 _]
      seq-local: [w1117 _ _ _] -> [_ _ w1280 _]
      seq-local: [w1116 _ _ _] -> [_ _ w1278 _]
      seq-local: [w1115 _ _ _] -> [_ _ w1277 _]
      tunnel: w1114 -> [w1126 _ _ _]
      tunnel: [_ _ _ w1310] -> w1104
      tunnel: [_ w1266 _ _] -> w1113
      tunnel: [_ _ w1285 _] -> w1112
      tunnel: w1111 -> [w1124 _ _ _]
      tunnel: [_ _ w1279 _] -> w1110
      tunnel: w1109 -> [w1123 _ _ _]
      tunnel: [_ _ w1281 _] -> w1108
      tunnel: [_ _ w1282 _] -> w1107
      tunnel: w1106 -> [w1119 _ _ _]
      frame #0 {
        # "Детектирование SEL"
        n591 = local read "P2 CH0"() -> (w1117:bool)
        n592 = local read "P1 CH1"() -> (w1116:bool)
        n593 = local read "P2 CH1"() -> (w1118:bool)
        n594 = flat-sequence {
          tunnel: w1121 -> [w1159]
          frame #0 {
            n595 = case shown="True" w1159 {
              frame False {
              }
              frame True {
                n596 = Wait (ms)(milliseconds to wait=u32 50) -> ()  [unwired: 1 out]
              }
            }
          }
          frame #1 {
            n597 = local read "P1CH1_cur, A"() -> (w1164:dbl)
            n598 = local read "SIM_SEL"() -> (w1162:bool)
            n599 = Greater Or Equal?(x=w1164, y="P1 CH1_selcur, A") -> (x >= y?=w1165:bool)
            n600 = Or(x=w1162, y=w1165) -> (x .or. y?=→"P1 CH1_warning":bool)
          }
          frame #2 {
            n601 = local read "Считать SIM_SEL"() -> (w1171:bool)
            n602 = local read "SIM_SEL"() -> (w1170:bool)
            n603 = local read "P1 CH1_warning"() -> (w1166:bool)
            n604 = Not(x=w1170) -> (.not. x?=w1169:bool)
            n605 = Select(t=TRUE, s=w1171, f=w1169) -> (s? t:f=w1167:bool)
            n606 = And(x=w1166, y=w1167) -> (x .and. y?=w1172:bool)
            n607 = case shown="True" w1172 {
              frame False {
              }
              frame True {
                n608 = local read "P1 CH1_counter"() -> (w1174:u32)
                n609 = Increment(x=w1174) -> (x+1=→"P1 CH1_counter":u32)
              }
            }
          }
        }
        n610 = flat-sequence {
          tunnel: w1122 -> [w1143]
          frame #0 {
            n611 = case shown="True" w1143 {
              frame False {
              }
              frame True {
                n612 = Wait (ms)(milliseconds to wait=u32 50) -> ()  [unwired: 1 out]
              }
            }
          }
          frame #1 {
            n613 = local read "P2 CH0_cur, A"() -> (w1149:dbl)
            n614 = local read "SIM_SEL"() -> (w1146:bool)
            n615 = Greater Or Equal?(x=w1149, y="P2 CH0_selcur, A") -> (x >= y?=w1148:bool)
            n616 = Or(x=w1146, y=w1148) -> (x .or. y?=→"P2 CH0_warning":bool)
          }
          frame #2 {
            n617 = local read "Считать SIM_SEL"() -> (w1153:bool)
            n618 = local read "SIM_SEL"() -> (w1154:bool)
            n619 = local read "P2 CH0_warning"() -> (w1150:bool)
            n620 = Not(x=w1154) -> (.not. x?=w1155:bool)
            n621 = Select(t=TRUE, s=w1153, f=w1155) -> (s? t:f=w1152:bool)
            n622 = And(x=w1150, y=w1152) -> (x .and. y?=w1151:bool)
            n623 = case shown="True" w1151 {
              frame False {
              }
              frame True {
                n624 = local read "P2 CH0_counter"() -> (w1158:u32)
                n625 = Increment(x=w1158) -> (x+1=→"P2 CH0_counter":u32)
              }
            }
          }
        }
        n626 = flat-sequence {
          tunnel: w1125 -> [w1175]
          frame #0 {
            n627 = case shown="True" w1175 {
              frame False {
              }
              frame True {
                n628 = Wait (ms)(milliseconds to wait=u32 50) -> ()  [unwired: 1 out]
              }
            }
          }
          frame #1 {
            n629 = local read "P1 CH0_cur, A"() -> (w1181:dbl)
            n630 = Greater Or Equal?(x=w1181, y="P1 CH0_selcur, A") -> (x >= y?=w1180:bool)
            n631 = Or(x="SIM_SEL", y=w1180) -> (x .or. y?=→"P1 CH0_warning":bool)
          }
          frame #2 {
            n632 = local read "SIM_SEL"() -> (w1187:bool)
            n633 = local read "P1 CH0_warning"() -> (w1182:bool)
            n634 = Not(x=w1187) -> (.not. x?=w1186:bool)
            n635 = Select(t=TRUE, s="Считать SIM_SEL", f=w1186) -> (s? t:f=w1183:bool)
            n636 = And(x=w1182, y=w1183) -> (x .and. y?=w1188:bool)
            n637 = case shown="True" w1188 {
              frame False {
              }
              frame True {
                n638 = local read "P1 CH0_counter"() -> (w1190:u32)
                n639 = Increment(x=w1190) -> (x+1=→"P1 CH0_counter":u32)
              }
            }
          }
        }
        n640 = flat-sequence {
          tunnel: w1120 -> [w1127]
          frame #0 {
            n641 = case shown="True" w1127 {
              frame False {
              }
              frame True {
                n642 = Wait (ms)(milliseconds to wait=u32 50) -> ()  [unwired: 1 out]
              }
            }
          }
          frame #1 {
            n643 = local read "P2 CH1_cur, A"() -> (w1131:dbl)
            n644 = local read "SIM_SEL"() -> (w1129:bool)
            n645 = Greater Or Equal?(x=w1131, y="P2 CH1_selcur, A") -> (x >= y?=w1132:bool)
            n646 = Or(x=w1129, y=w1132) -> (x .or. y?=→"P2 CH1_warning":bool)
          }
          frame #2 {
            n647 = local read "Считать SIM_SEL"() -> (w1140:bool)
            n648 = local read "SIM_SEL"() -> (w1139:bool)
            n649 = local read "P2 CH1_warning"() -> (w1134:bool)
            n650 = Not(x=w1139) -> (.not. x?=w1138:bool)
            n651 = Select(t=TRUE, s=w1140, f=w1138) -> (s? t:f=w1136:bool)
            n652 = And(x=w1134, y=w1136) -> (x .and. y?=w1135:bool)
            n653 = case shown="True" w1135 {
              frame False {
              }
              frame True {
                n654 = local read "P2 CH1_counter"() -> (w1142:u32)
                n655 = Increment(x=w1142) -> (x+1=→"P2 CH1_counter":u32)
              }
            }
          }
        }
        n656 = local read "P1 CH0"() -> (w1115:bool)
        n657 = Greater?(x=w1117, y=w1123) -> (0:w1122:bool)
        n658 = Greater?(x=w1115, y=w1126) -> (0:w1125:bool)
        n659 = Greater?(x=w1116, y=w1124) -> (0:w1121:bool)
        n660 = Greater?(x=w1118, y=w1119) -> (0:w1120:bool)
      }
      frame #1 {
        w1193 = "\t"
        w1205 = "\t"
        w1207 = "\t"
        w1209 = "\t"
        w1194 = "\t"
        w1195 = "\t"
        w1196 = "\t"
        w1197 = "\t"
        w1240 = 0
        w1239 = 6
        w1235 = 6
        w1245 = 0
        w1246 = 6
        w1250 = 6
        w1259 = 0
        w1258 = 6
        w1253 = 6
        w1262 = 0
        w1263 = 6
        w1269 = 6
        # "Запись логов"
        n661 = local read "P2 CH1, V"() -> (w1242:dbl)
        n662 = local read "P2 CH1_cur, A"() -> (w1238:dbl)
        n663 = local read "P2 CH1_counter"() -> (w1241:u32)
        n664 = local read "P2 CH1_warning"() -> (w1237:bool)
        n665 = local read "P1 CH0, V"() -> (w1267:dbl)
        n666 = local read "P1 CH0_cur, A"() -> (w1264:dbl)
        n667 = local read "P1 CH0_counter"() -> (w1261:u32)
        n668 = local read "P1 CH0_warning"() -> (w1265:bool)
        n669 = local read "P1 CH1, V"() -> (w1255:dbl)
        n670 = local read "P1CH1_cur, A"() -> (w1257:dbl)
        n671 = local read "P1 CH1_counter"() -> (w1260:u32)
        n672 = local read "P1 CH1_warning"() -> (w1256:bool)
        n673 = local read "P2 CH0, V"() -> (w1243:dbl)
        n674 = local read "P2 CH0_cur, A"() -> (w1247:dbl)
        n675 = local read "P2 CH0_counter"() -> (w1244:u32)
        n676 = local read "P2 CH0_warning"() -> (w1248:bool)
        n677 = Number To Fractional String(number=w1242, width (-)=w1235, precision (6)=w1235) -> (F-format string=w1221:string)  [unwired: 1 in]
        n678 = Number To Fractional String(number=w1238, width (-)=w1239, precision (6)=w1239) -> (F-format string=w1220:string)  [unwired: 1 in]
        n679 = Number To Fractional String(number=w1241, width (-)=w1240, precision (6)=w1240) -> (F-format string=w1219:string)  [unwired: 1 in]
        n680 = Number To Fractional String(number=w1267, width (-)=w1269, precision (6)=w1269) -> (F-format string=w1233:string)  [unwired: 1 in]
        n681 = Number To Fractional String(number=w1264, width (-)=w1263, precision (6)=w1263) -> (F-format string=w1232:string)  [unwired: 1 in]
        n682 = Number To Fractional String(number=w1261, width (-)=w1262, precision (6)=w1262) -> (F-format string=w1231:string)  [unwired: 1 in]
        n683 = Number To Fractional String(number=w1255, width (-)=w1253, precision (6)=w1253) -> (F-format string=w1229:string)  [unwired: 1 in]
        n684 = Number To Fractional String(number=w1257, width (-)=w1258, precision (6)=w1258) -> (F-format string=w1228:string)  [unwired: 1 in]
        n685 = Number To Fractional String(number=w1260, width (-)=w1259, precision (6)=w1259) -> (F-format string=w1227:string)  [unwired: 1 in]
        n686 = Number To Fractional String(number=w1243, width (-)=w1250, precision (6)=w1250) -> (F-format string=w1225:string)  [unwired: 1 in]
        n687 = Number To Fractional String(number=w1247, width (-)=w1246, precision (6)=w1246) -> (F-format string=w1224:string)  [unwired: 1 in]
        n688 = Number To Fractional String(number=w1244, width (-)=w1245, precision (6)=w1245) -> (F-format string=w1223:string)  [unwired: 1 in]
        n689 = Select(t="!!!3", s=w1237, f="") -> (s? t:f=w1218:string)
        n690 = Select(t="!!!0", s=w1265, f="") -> (s? t:f=w1230:string)
        n691 = Select(t="!!!1", s=w1256, f="") -> (s? t:f=w1226:string)
        n692 = Select(t="!!!2", s=w1248, f="") -> (s? t:f=w1222:string)
        n693 = local read "P1 CH0 Used"() -> (w1214:bool)
        n694 = local read "P1 CH1 Used"() -> (w1213:bool)
        n695 = local read "P2 CH0 Used"() -> (w1212:bool)
        n696 = local read "P2 CH1 Used"() -> (w1211:bool)
        n697 = Concatenate Strings(w1197, w1233, w1197, w1232, w1197, w1231, w1197, w1230) -> (w1216:string)
        n698 = Concatenate Strings(w1196, w1229, w1196, w1228, w1196, w1227, w1196, w1226) -> (w1217:string)
        n699 = Concatenate Strings(w1195, w1225, w1195, w1224, w1195, w1223, w1195, w1222) -> (w1215:string)
        n700 = Concatenate Strings(w1194, w1221, w1194, w1220, w1194, w1219, w1194, w1218) -> (w1210:string)
        n701 = Concatenate Strings(w1209, w1209, w1209, w1209) -> (w1208:string)
        n702 = Concatenate Strings(w1207, w1207, w1207, w1207) -> (w1206:string)
        n703 = Concatenate Strings(w1205, w1205, w1205, w1205) -> (w1204:string)
        n704 = Concatenate Strings(w1193, w1193, w1193, w1193) -> (w1203:string)
        n705 = Select(t=w1216, s=w1214, f=w1208) -> (s? t:f=w1202:string)
        n706 = Select(t=w1217, s=w1213, f=w1206) -> (s? t:f=w1201:string)
        n707 = Select(t=w1215, s=w1212, f=w1204) -> (s? t:f=w1200:string)
        n708 = Select(t=w1210, s=w1211, f=w1203) -> (s? t:f=w1199:string)
        n709 = Get Date/Time In Seconds() -> (seconds since 1Jan1904=w1272:timestamp)
        n710 = Format Date/Time String(time format string (%c)="%H:%M:%S:%3u", seconds (now)=w1272) -> (date/time string=w1270:string)  [unwired: 1 in]
        n711 = local read "SEL output file refnum"() -> (w1191:refnum<file>)
        n712 = Concatenate Strings(w1270, w1202, w1201, w1200, w1199, "\r\n") -> (w1198:string)
        n713 = Format Into String(initial string=w1191, w1198) -> (resulting string=w1266:refnum<file>)  [unwired: 2 in, 1 out]
      }
      frame #2 {
        n714 = local read "P1 CH0_warning"() -> (w1284:bool)
        "SEL" <- w1284
        n715 = local read "P1 CH1_warning"() -> (w1276:bool)
        n716 = local read "P2 CH0_warning"() -> (w1274:bool)
        n717 = local read "P2 CH1_warning"() -> (w1275:bool)
        n718 = local write "SEL"(w1274) -> ()
        n719 = local write "SEL"(w1276) -> ()
        n720 = local write "SEL"(w1275) -> ()
        n721 = case shown="True" w1284 {
          tunnel: [w1304 w1305] -> w1285
          tunnel: w1277 -> [w1304 _]
          frame False {
          }
          frame True {
            n722 = flat-sequence {
              tunnel: [FALSE] -> w1305
              frame #0 {
                n723 = local write "P1 CH0"(FALSE ("Power")) -> ()
              }
              frame #1 {
                n724 = Wait (ms)(milliseconds to wait=u32 100 ("Wait_parry, ms")) -> ()  [unwired: 1 out]
              }
              frame #2 {
                n725 = local write "P1 CH0"(TRUE ("Power")) -> ()
              }
            }
          }
        }
        n726 = case shown="True" w1276 {
          tunnel: [w1298 w1299] -> w1279
          tunnel: w1278 -> [w1298 _]
          frame False {
          }
          frame True {
            n727 = flat-sequence {
              tunnel: [FALSE] -> w1299
              frame #0 {
                n728 = local write "P1 CH1"(FALSE ("Power")) -> ()
              }
              frame #1 {
                n729 = Wait (ms)(milliseconds to wait=u32 100 ("Wait_parry, ms")) -> ()  [unwired: 1 out]
              }
              frame #2 {
                n730 = local write "P1 CH1"(TRUE ("Power")) -> ()
              }
            }
          }
        }
        n731 = case shown="True" w1274 {
          tunnel: [w1292 w1293] -> w1281
          tunnel: w1280 -> [w1292 _]
          frame False {
          }
          frame True {
            n732 = flat-sequence {
              tunnel: [FALSE] -> w1293
              frame #0 {
                n733 = local write "P2 CH0"(FALSE ("Power")) -> ()
              }
              frame #1 {
                n734 = Wait (ms)(milliseconds to wait=u32 100 ("Wait_parry, ms")) -> ()  [unwired: 1 out]
              }
              frame #2 {
                n735 = local write "P2 CH0"(TRUE ("Power")) -> ()
              }
            }
          }
        }
        n736 = case shown="True" w1275 {
          tunnel: [w1286 w1287] -> w1282
          tunnel: w1283 -> [w1286 _]
          frame False {
          }
          frame True {
            n737 = flat-sequence {
              tunnel: [FALSE] -> w1287
              frame #0 {
                n738 = local write "P2 CH1"(FALSE ("Power")) -> ()
              }
              frame #1 {
                n739 = Wait (ms)(milliseconds to wait=u32 100 ("Wait_parry, ms")) -> ()  [unwired: 1 out]
              }
              frame #2 {
                n740 = local write "P2 CH1"(TRUE ("Power")) -> ()
              }
            }
          }
        }
      }
      frame #3 {
        n741 = local read "STOP"() -> (w1310:bool)
      }
    }
  }
  n742 = flat-sequence {
    tunnel: w30 -> [w1324]
    tunnel: w25 -> [w1323]
    tunnel: w24 -> [w1322]
    tunnel: w21 -> [_]
    tunnel: w20 -> [w1321]
    tunnel: w19 -> [w1320]
    frame #0 {
      # "STOP"
      n743 = call <instrlib>:"niDCPower Close.vi"("error in (no error)"=w1320, "instrument handle"=w1322) -> ("error out"=w1318:errorcluster)  [unwired: 9 in]
      n744 = call <instrlib>:"niDCPower Close.vi"("error in (no error)"=w1321, "instrument handle"=w1323) -> ("error out"=w1319:errorcluster)  [unwired: 9 in]
      n745 = Close File(refnum=w1324) -> ()  [unwired: 1 in, 2 out]
      n746 = call <vilib>:"Simple Error Handler.vi"("error in (no error)"=w1318) -> ("error out"=w1316:errorcluster)  [unwired: 1 in, 7 out]
      n747 = local write "DC Power 2 error out"(w1316) -> ()
      n748 = call <vilib>:"Simple Error Handler.vi"("error in (no error)"=w1319) -> ("error out"=w1317:errorcluster)  [unwired: 1 in, 7 out]
      n749 = local write "DC Power 1 error out"(w1317) -> ()
      n750 = Wait (ms)(milliseconds to wait=u32 1) -> ()  [unwired: 1 out]
      n751 = property on="NI DMM 1 Tab" class="TabCtl (strict)"("DisabledEnum"=T3."Enabled" ("Disabled")) -> ()  [unwired: 2 in, 2 out]
      n752 = property on="NI DMM 2 Tab" class="TabCtl (strict)"("DisabledEnum"=T3."Enabled" ("Disabled")) -> ()  [unwired: 2 in, 2 out]
      n753 = property on="Ophir 1 Tab" class="TabCtl (strict)"("DisabledEnum"=T3."Enabled" ("Disabled")) -> ()  [unwired: 2 in, 2 out]
      n754 = property on="Ophir 2 Tab" class="TabCtl (strict)"("DisabledEnum"=T3."Enabled" ("Disabled")) -> ()  [unwired: 2 in, 2 out]
      n755 = property on="NI Scope Tab" class="TabCtl (strict)"("DisabledEnum"=T3."Enabled" ("Disabled")) -> ()  [unwired: 2 in, 2 out]
    }
  }
  n756 = case shown="True" w2 {
    tunnel: w3 -> [_ w1327]
    frame False {
    }
    frame True {
      n757 = local read "Ophir 2 dup Visa Session"() -> (w1329:refnum<visa-resource-name>)
      n758 = local read "Ophir 2 error out"() -> (w1328:errorcluster)
      n759 = while {
        tunnel: [w1340] -> w1331
        tunnel: [w1334] -> w1330
        tunnel: w1329 -> [w1338]
        tunnel: w1328 -> [w1337]
        tunnel: w1327 -> [_]
        shift-right: [w1335] -> _
        shift-left: 0.0 -> [w1336]
        stop <- w1339 stop-if-true
        n760 = Wait (ms)(milliseconds to wait="Ophir 2 Wait") -> ()  [unwired: 1 out]
        n761 = stacked-sequence {
          tunnel: [w1356] -> w1340
          tunnel: [w1341] -> w1339
          tunnel: w1338 -> [w1342]
          tunnel: w1337 -> [w1351]
          tunnel: w1336 -> [w1345]
          tunnel: [w1343] -> w1335
          tunnel: [w1342] -> w1334
          frame #0 {
            n762 = Fract/Exp String To Number(string="Ophir 2 units") -> (number=w1344:dbl)  [unwired: 3 in, 1 out]
            n763 = call "Ophir SendPower.vi"("Visa Session"=w1342, "error in (no error)"=w1351) -> ("Value Number"=w1353:dbl, "Value String"=w1354:string, "error out"=w1356:errorcluster)  [unwired: 1 out]
            "Ophir 2 Real Optical Power" <- w1353
            n764 = call "Ophir Over.vi"("Value String"=w1354) -> ("Overrange"=→"Ophir 2 Over Range":bool)
            n765 = Multiply(x=w1353, y=w1344) -> (x*y=w1349:dbl)
            "Ophir 2 Char" <- w1349
            "Ophir 2 Optical Power" <- w1349
            n766 = Greater Or Equal?(x=w1349, y=w1345) -> (x >= y?=w1350:bool)
            n767 = Select(t=0.0, s="Ophir 2 Clear", f=w1345) -> (s? t:f=w1348:dbl)
            n768 = Select(t=w1349, s=w1350, f=w1348) -> (s? t:f=w1343:dbl)
            "Ophir 2 MAX" <- w1343
            n769 = local read "STOP"() -> (w1341:bool)
          }
        }
      }
      n770 = VISA Close(VISA resource name=w1330, error in (no error)=w1331) -> (error out=w1332:errorcluster)
      n771 = call "Ophir Error Message.vi"("error in (no error)"=w1332) -> ()  [unwired: 3 in, 4 out]
    }
  }
  n772 = case shown="True" w6 {
    tunnel: w3 -> [_ w1358]
    frame False {
    }
    frame True {
      n773 = local read "Ophir 1 dup Visa Session"() -> (w1360:refnum<visa-resource-name>)
      n774 = local read "Ophir 1 error out"() -> (w1359:errorcluster)
      n775 = while {
        tunnel: [w1371] -> w1362
        tunnel: [w1365] -> w1361
        tunnel: w1360 -> [w1369]
        tunnel: w1359 -> [w1368]
        tunnel: w1358 -> [_]
        shift-right: [w1366] -> _
        shift-left: 0.0 -> [w1367]
        stop <- w1370 stop-if-true
        n776 = Wait (ms)(milliseconds to wait="Ophir 1 Wait") -> ()  [unwired: 1 out]
        n777 = stacked-sequence {
          tunnel: [w1387] -> w1371
          tunnel: [w1372] -> w1370
          tunnel: w1369 -> [w1374]
          tunnel: w1368 -> [w1383]
          tunnel: w1367 -> [w1377]
          tunnel: [w1375] -> w1366
          tunnel: [w1374] -> w1365
          frame #0 {
            n778 = Fract/Exp String To Number(string="Ophir 1 units") -> (number=w1376:dbl)  [unwired: 3 in, 1 out]
            n779 = call "Ophir SendPower.vi"("Visa Session"=w1374, "error in (no error)"=w1383) -> ("Value Number"=w1373:dbl, "Value String"=w1385:string, "error out"=w1387:errorcluster)  [unwired: 1 out]
            "Ophir 1 Real Optical Power" <- w1373
            n780 = call "Ophir Over.vi"("Value String"=w1385) -> ("Overrange"=→"Ophir 1 Over Range":bool)
            n781 = Multiply(x=w1373, y=w1376) -> (x*y=w1381:dbl)
            "Ophir 1 Char" <- w1381
            "Ophir 1 Optical Power" <- w1381
            n782 = Greater Or Equal?(x=w1381, y=w1377) -> (x >= y?=w1382:bool)
            n783 = Select(t=0.0, s="Ophir 1 Clear", f=w1377) -> (s? t:f=w1380:dbl)
            n784 = Select(t=w1381, s=w1382, f=w1380) -> (s? t:f=w1375:dbl)
            "Ophir 1 MAX" <- w1375
            n785 = local read "STOP"() -> (w1372:bool)
          }
        }
      }
      n786 = VISA Close(VISA resource name=w1361, error in (no error)=w1362) -> (error out=w1363:errorcluster)
      n787 = call "Ophir Error Message.vi"("error in (no error)"=w1363) -> ()  [unwired: 3 in, 4 out]
    }
  }
